vi "Retrieve and visualize_SE.vi"(11 "Field/Temperature":i32(slide) min=0 max=36 step=1 scale=-1.1..1.0) -> (1 "slowest":dbl=-2499.957 format="%#_6p")   [LabVIEW 2020, in "Retrieve and Visualize.lvclass"]
uses:
  Retrieve and Visualize.lvclass
  <vilib>/Analysis/NI_AAL_SigProc.lvlib
  <userlib>/LevyLab/Graph Utilities/graph_utilities.lvclass
  <userlib>/LevyLab/XY Utilities/xy_utilities.lvlib
  <userlib>/LevyLab/XY Utilities/subVIs/Interpolate (single).vi
  <userlib>/LevyLab/XY Utilities/Typedefs/Interpolation Configuration--cluster.ctl
  <userlib>/LevyLab/LV-Data/LV-Data.ITX/LV-Data.ITX.lvclass
  <userlib>/LevyLab/Instrument Framework/SMOs/Configuration/Configuration.lvclass
  typedefs/Choose Intensity Data--enum.ctl
  typedefs/INI--Cluster.ctl
  <vilib>/Utility/sysdir.llb/System Directory Type.ctl
  <userlib>/_OpenG.lib/file/file.llb/File Exists - Scalar__ogtk.vi
  typedefs/IV Setup--Cluster.ctl
  <userlib>/LevyLab/LV-Data/LV-Data/Typedefs/File Type--enum.ctl
  <userlib>/LevyLab/LV-Data/LV-Data/LV-Data.lvclass
panel:
  in  "Window [h] (2)":dbl=2.0
  in  "Interval Units (points)":enum16{"Points", "Data"}(ring)
  in  "Subset Slider (%)":cluster{dbl, dbl}(slide)={75.0, 25.0} scale=0.0..100.0 scale format="%#_6f"
  in  "Export ITX Name":string="B2"
  in  "Export What?":T1(ring)
  in  "Export ITX":bool
  in  "Export ITX Path":path=path "C:/"
  out "Status":string="Exit"
  out "Slow":dbl=88828.125
  out "Fast":dbl=-0.009836065573770498
  in  "OK":bool
  in  "Open DAT Path":path=path "C:/"
  in  "S-G side points (4T)":i32=8
  in  "S-G side points (2T)":i32=12
  in  "Visualize Button":bool
  in  "Tab Control":T2(tab)=enum."Intensity Graphs"
  out "Comments":string
  in  "Check Files Button":bool
  in  "Generate Button":bool
  in  "Additional comments":string
  in  "Field Period":i32=1
  in  "# of fields/Temperatures":i32=1
  in  "Path":path=path "C:/"
  in  "DAT folder":path=path "C:/"
  in  "IV file name":string="Name.dat"
  in  "IV setup":T3={"# Vslow"=11, "# Vfast"=251, "#IV Curves at each gate"=1, "B/T offset"=0, "Discard first # curves"=0, "Manual offset"=0}
  in  "Scan names":string[](array[string])=["appliedVsg", "appliedField", "appliedField"]
  in  "Portion of data (%)":cluster{dbl, dbl}(slide)={1.0, 0.0} scale=0.0..100.0
  in  "Decimate point":dbl=10.0 format="%#_1f"
  in  "Extract paramaters from comments?":bool=TRUE
  in  "index":T4={"A"=7, "B"=6, "C"=3, "D"=6, "E"=3, "N1"=2, "N2"=2, "N3"=3, "N4"=4, "A 1"=8, "A 2"=10, "C 1"=5, "C 2"=1, "E 2"=4}
  in  "T/B third axis":bool
  in  "File Type":T5
  out "IV":cluster{dbl[], dbl[]}[](graph)
  out "dI/dV":cluster{dbl[], dbl[]}[](graph)
  out "dI/dV 2T":cluster{dbl[], dbl[]}[](graph)
  out "IV 2T":cluster{dbl[], dbl[]}[](graph)
  out "dV/dI":cluster{dbl[], dbl[]}[](graph)
  out "dV/dI 2T":cluster{dbl[], dbl[]}[](graph)
  out "IV slow 2T":cluster{dbl[], dbl[]}[](graph)
  out "dI/dV slow 2T":cluster{dbl[], dbl[]}[](graph)
  out "IV slow 4T":cluster{dbl[], dbl[]}[](graph)
  out "dI/dV slow 4T":cluster{dbl[], dbl[]}[](graph)
  out "IV vary 3rd 2T":cluster{dbl[], dbl[]}[](graph)
  out "dI/dV vary 3rd 2T":cluster{dbl[], dbl[]}[](graph)
  out "IV vary 3rd 4T":cluster{dbl[], dbl[]}[](graph)
  out "dI/dV vary 3rd 4T":cluster{dbl[], dbl[]}[](graph)
  in  "fake point 1":dbl format="%#_6p"
  in  "Log scale? 1":bool
  in  "e^2/h? 1":bool=TRUE
  in  "e^2/h? 2":bool=TRUE
  in  "Log scale? 2":bool
  in  "fake point 2":dbl format="%#_6p"
  in  "Intensity 1":T6=enum."G-4T"
  out "Intensity Graph 1":dbl[][](graph)
  out "Intensity Graph 2":dbl[][](graph)
  out "H Cut 1":cluster{dbl[], dbl[]}[](graph)
  out "V Cut 1":cluster{dbl[], dbl[]}[](graph)
  out "H Cut 2":cluster{dbl[], dbl[]}[](graph)
  out "V Cut 2":cluster{dbl[], dbl[]}[](graph)
  in  "Intensity 2":T6=enum."dGdVsg-4T"
  in  "X Offset 1":dbl format="%#_6p"
  in  "X Offset 2":dbl format="%#_6p"
  out "x3D Intensity Graph 11":dbl[][](graph)
  out "x3D Intensity Graph 10":dbl[][](graph)
  out "x3D Intensity Graph 9":dbl[][](graph)
  out "x3D Transconductance 2":dbl[][](graph)
  out "bottom loop":dbl[](graph)
  out "xalpha top loop":dbl[](graph)
  out "xalpha Top loop Intensity Graph":dbl[][](graph)
  out "xalpha Vsd vs Vsg":cluster{dbl[], dbl[]}(graph)
  in  "xalpha threshold 2":dbl format="%0.2f"
  in  "xalpha width 2":i32=3 min=3
  out "xalpha Y line cut 9":cluster{dbl[], dbl[]}[](graph)
  out "xalpha Vsg?":dbl[](array[numeric])
  out "xalpha vertical peak diff":dbl[](array[numeric])
  in  "xalpha threshold":dbl format="%0.2f"
  in  "xalpha width":i32=3 min=3
  in  "xalpha derivative bin size":dbl=10.0
  in  "Diff Interval":dbl=12.0
  in  "derivative bin size 2":dbl=12.0
  in  "derivative bin size 1":dbl=12.0
  in  "SG Filter?":bool=TRUE
  out "Cursor Graph":cluster{dbl[], dbl[]}(graph)
  # "I+"
  # "V+"
  # "Vsg1"
  # "Vsgw"
  # "Vsg2"
  # "V-"
  # "I-"
  # "Input"
  # "Process Parameters"
  # "Vfast"
  # "Vslow"
  # "Vslowest"
  # "obsolete?"
  # "A: V4\nB: I\nC: V2\nD: I\nA1,A2: V4 SE\nC1,C2: V2 SE\n\n#todo: replace with rings"
  # "DOESN'T WORK ANY MORE"
  # "Output"
  # "#todo: add button to automatically populate output and filename fields"
  # "Used??"
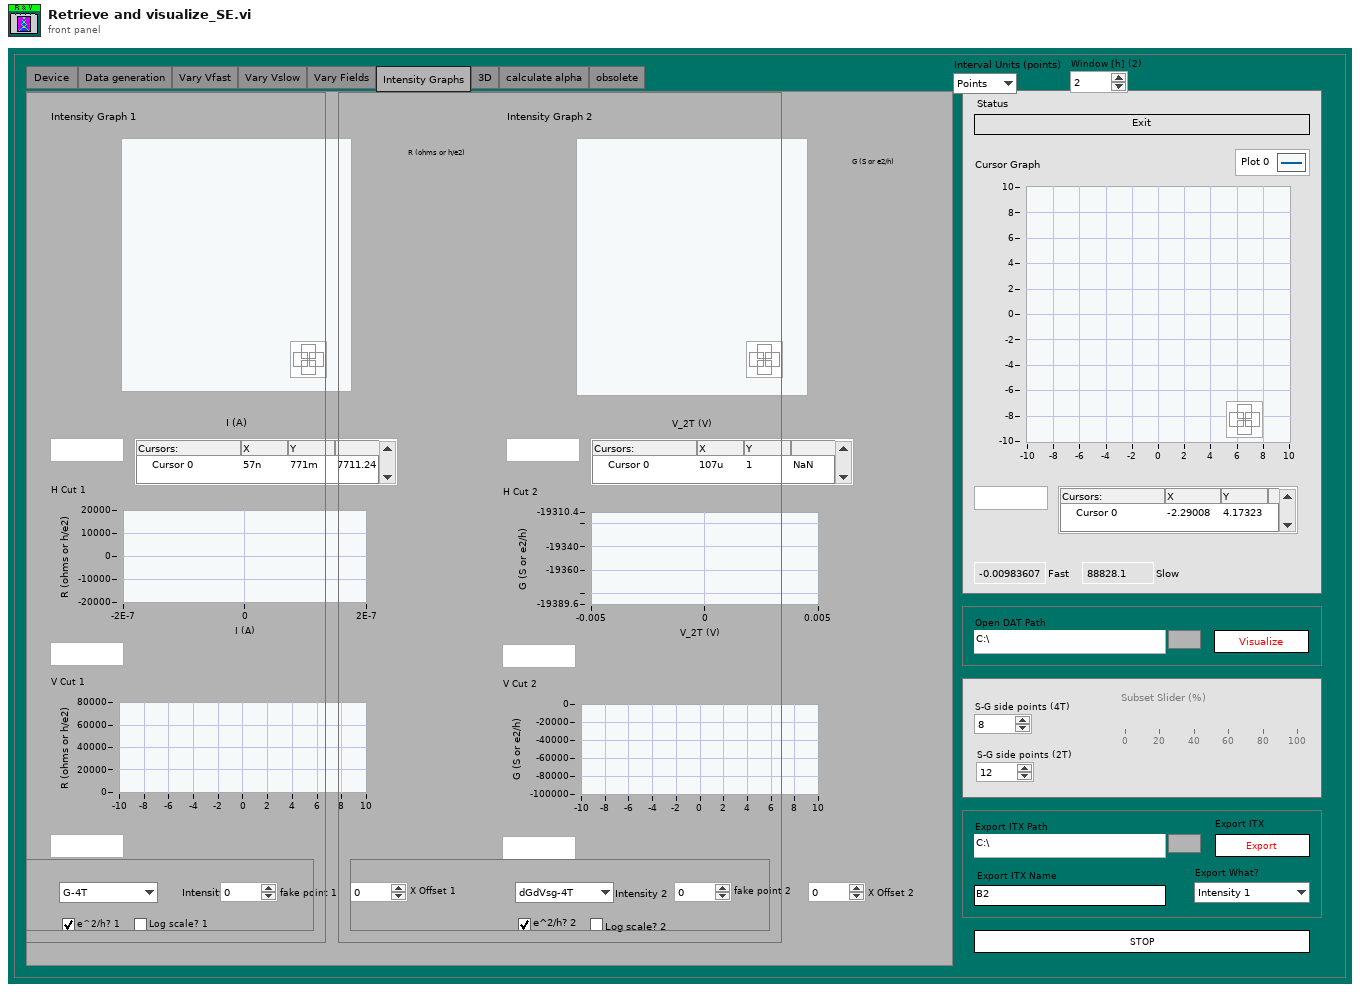
[diagram p1: front panel]
types:
  T1 = enum16{"Intensity 1", "H Cut 1", "V Cut 1", "Intensity 2", "H Cut 2", "V Cut 2"}
  T2 = enum32{"Device ", "Data generation", "Vary Vfast", "Vary Vslow", "Vary Fields", "Intensity Graphs", "3D", "calculate alpha", "obsolete"}
  T3 = typedef "Retrieve and Visualize.lvclass/IV Setup--Cluster.ctl" = cluster{"# Vslow":i32, "# Vfast":i32, "#IV Curves at each gate":i32, "B/T offset":i32, "Discard first # curves":i32, "Manual offset":i32}
  T4 = cluster{"A":i32, "B":i32, "C":i32, "D":i32, "E":i32, "N1":i32, "N2":i32, "N3":i32, "N4":i32, "A 1":i32, "A 2":i32, "C 1":i32, "C 2":i32, "E 2":i32}
  T5 = typedef "LV-Data.lvclass/File Type--enum.ctl" = enum16{"DAT", "ITX", "TDMS", "VI"}
  T6 = typedef "Retrieve and Visualize.lvclass/Choose Intensity Data--enum.ctl" = enum16{"IV-4T", "IV-2T", "R-4T", "G-4T", "R-2T", "G-2T", "dGdVsg-4T", "dGdVsg-2T"}
  T7 = enum32{"Device ", "Data generation", "Vary Vfast", "Vary Vslow", "Vary Fields", "Intensity Graphs", "3D (disabled)", "calculate alpha (disabled)"}
  T8 = cluster{"IV-4T":refnum<data-value>, "G-2T":refnum<data-value>, "R-2T":refnum<data-value>, "G-4T":refnum<data-value>, "R-4T":refnum<data-value>, "IV-2T":refnum<data-value>, "Vfast":dbl[][], "Vslow":dbl[], "Vslowest":dbl[], "Scan Names":string[]}
  T9 = typedef "xy_utilities.lvlib/Interpolation Configuration--cluster.ctl" = cluster{"X Low":dbl, "X High":dbl, "X Step":dbl, "Fake Point":dbl}
  T10 = typedef "LVOffsetAndMultiplierTypeDef.ctl" = cluster{"Offset":dbl, "Multiplier":dbl}
  T11 = enum32{"Invalid", "Standard", "Closed", "Hidden", "Minimized", "Maximized"}
  T12 = enum32{"invalid app kind", "Development System", "Run Time System", "Student Edition", "Embedded LabVIEW", "Evaluation", "Custom"}
  T13 = enum32{"Device ", "Data generation", "Vary Vfast", "Vary Vslow", "Vary Fields", "Intensity Graphs", "3D", "calculate alpha"}
  T14 = cluster{"V2T":string, "V+":string, "V-":string, "I (A)":string, "+X":string, "+Y":string, "-X":string, "-Y":string, "B":string}
  T15 = typedef "Retrieve and Visualize.lvclass/INI--Cluster.ctl" = cluster{"Open DAT Path":path, "Export ITX Path":path, "Export ITX Name":string, "Intensity 1":T6, "X Offset 1":dbl, "derivative bin size 1":dbl, "e^2/h? 1":bool, "Log scale? 1":bool, "fake point 1":dbl, "Intensity 2":T6, "X Offset 2":dbl, "derivative bin size 2":dbl, "e^2/h? 2":bool, "Log scale? 2":bool, "fake point 2":dbl}
  T16 = cluster{"Core":cluster{"Current VI Reference":refnum<vi>, "Close Panel on Exit?":bool}, "Retrieve and Visualize":refnum<class "Retrieve and Visualize.lvclass">, "Configuration":refnum<class "Configuration.lvclass">, "INI":T15, "DVR":cluster{"IV-4T":refnum<data-value>, "IV-2T":refnum<data-value>, "G-4T":refnum<data-value>, "R-4T":refnum<data-value>, "G-2T":refnum<data-value>, "R-2T":refnum<data-value>}, "Graph":cluster{"Intensity 1":refnum<class "graph_utilities.lvclass">, "V 1":refnum<class "graph_utilities.lvclass">, "H 1":refnum<class "graph_utilities.lvclass">, "Intensity 2":refnum<class "graph_utilities.lvclass">, "V 2":refnum<class "graph_utilities.lvclass">, "H 2":refnum<class "graph_utilities.lvclass">}, "Vfast":dbl[][], "Vslow":dbl[], "Vslowest":dbl[], "Scan Names":string[], "Vfast Slice":dbl[], "Vslow Slice":dbl[], "Page":i32, "Row Array":i32[], "Column Array":i32[], "Row":i32, "Column":i32}
  T17 = cluster{"Intensity 1":refnum<class "graph_utilities.lvclass">, "V 1":refnum<class "graph_utilities.lvclass">, "H 1":refnum<class "graph_utilities.lvclass">, "Intensity 2":refnum<class "graph_utilities.lvclass">, "V 2":refnum<class "graph_utilities.lvclass">, "H 2":refnum<class "graph_utilities.lvclass">}
  T18 = cluster{"IV-4T":refnum<data-value>, "IV-2T":refnum<data-value>, "G-4T":refnum<data-value>, "R-4T":refnum<data-value>, "G-2T":refnum<data-value>, "R-2T":refnum<data-value>}
  T19 = cluster{"Current VI Reference":refnum<vi>, "Close Panel on Exit?":bool}
  T20 = typedef "System Directory Type.ctl" = i32
  T21 = typedef "LVPointDoubleTypeDef.ctl" = cluster{"X":dbl, "Y":dbl}
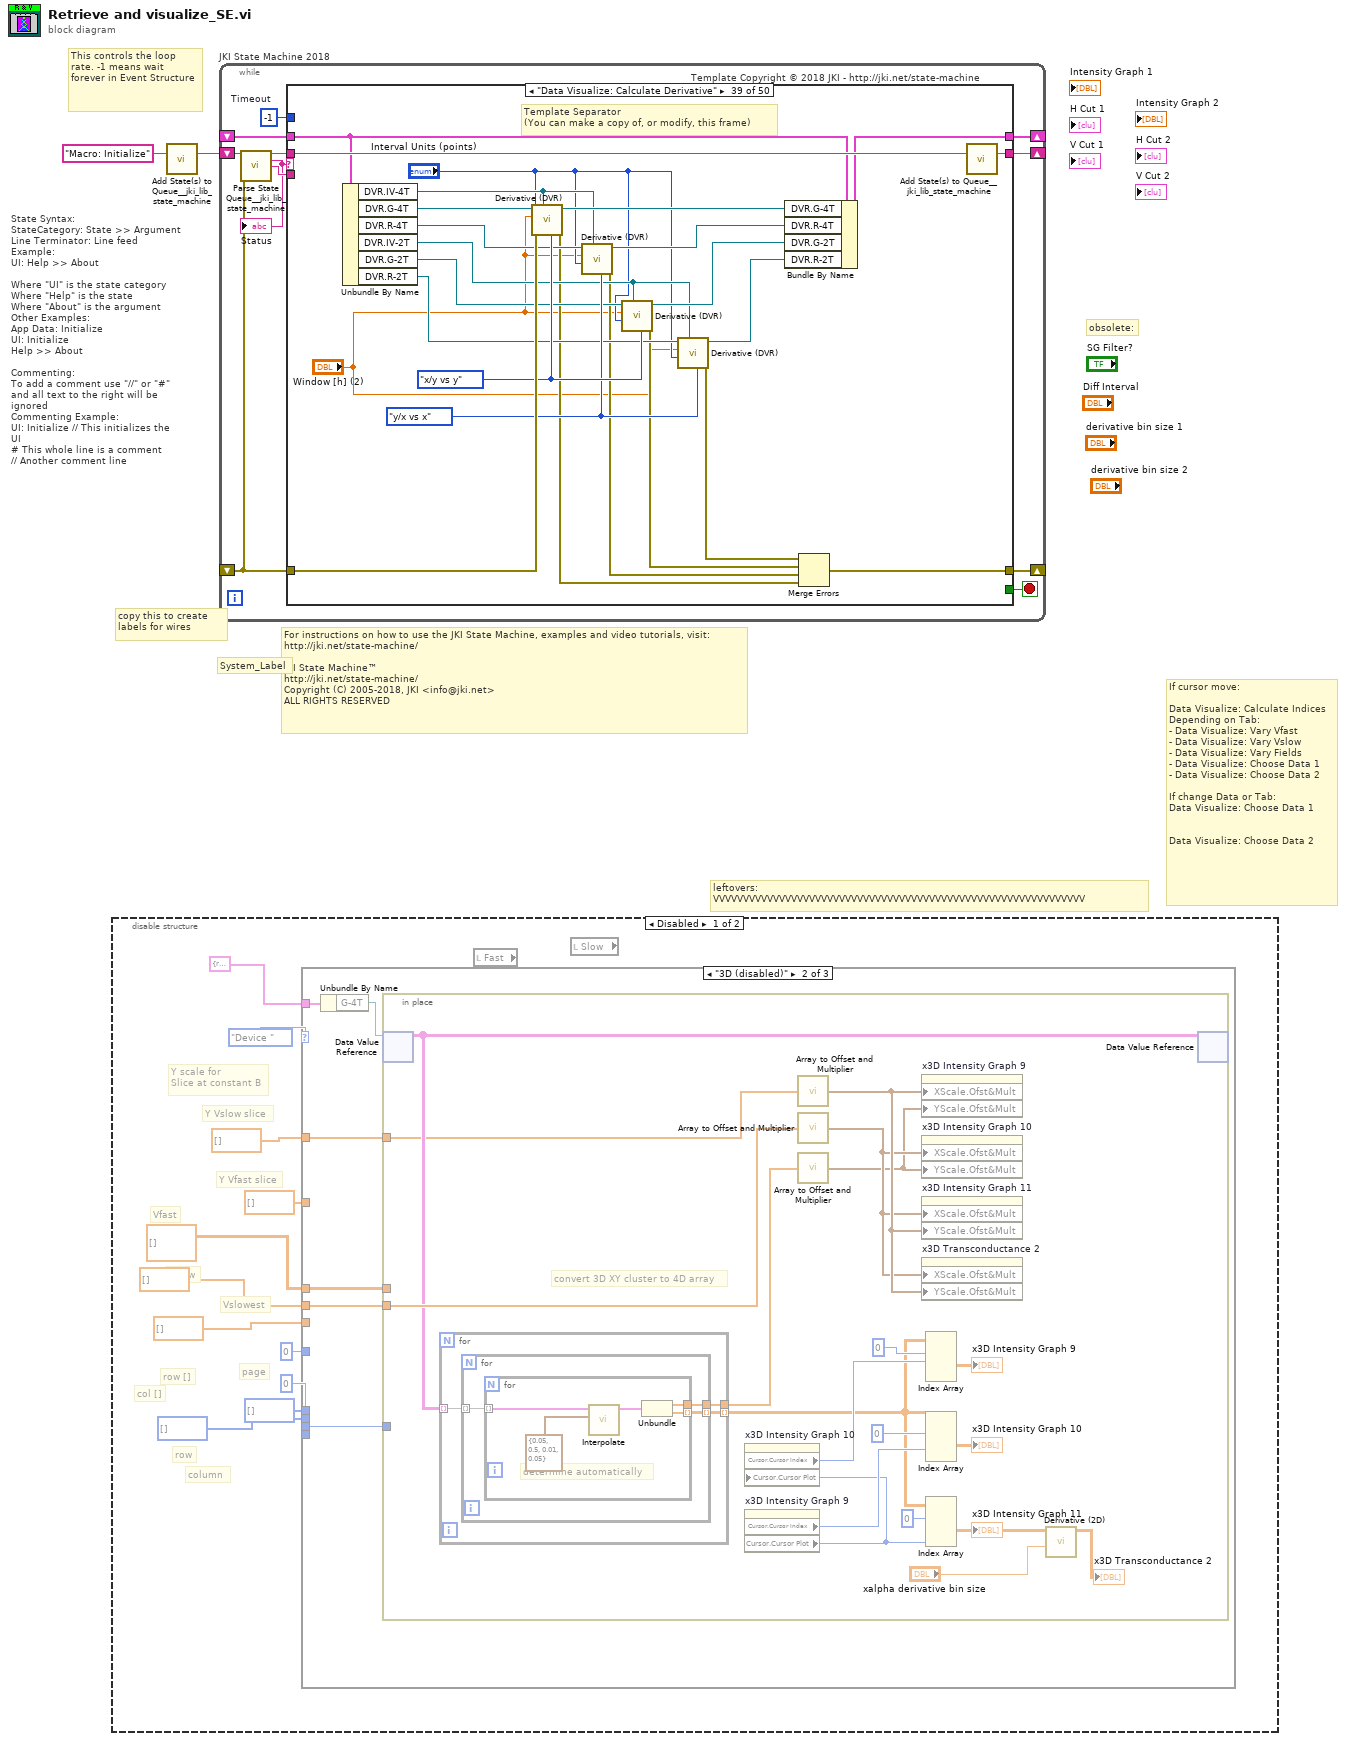
[diagram p0: block diagram]
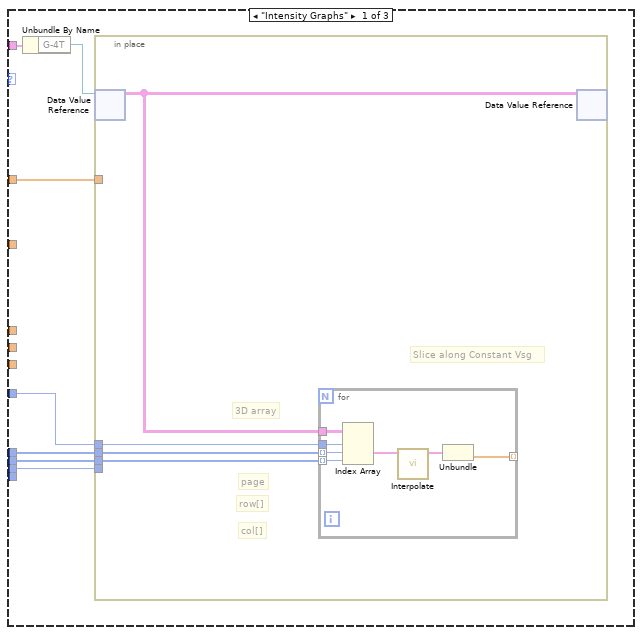
[diagram p2: hidden frame]
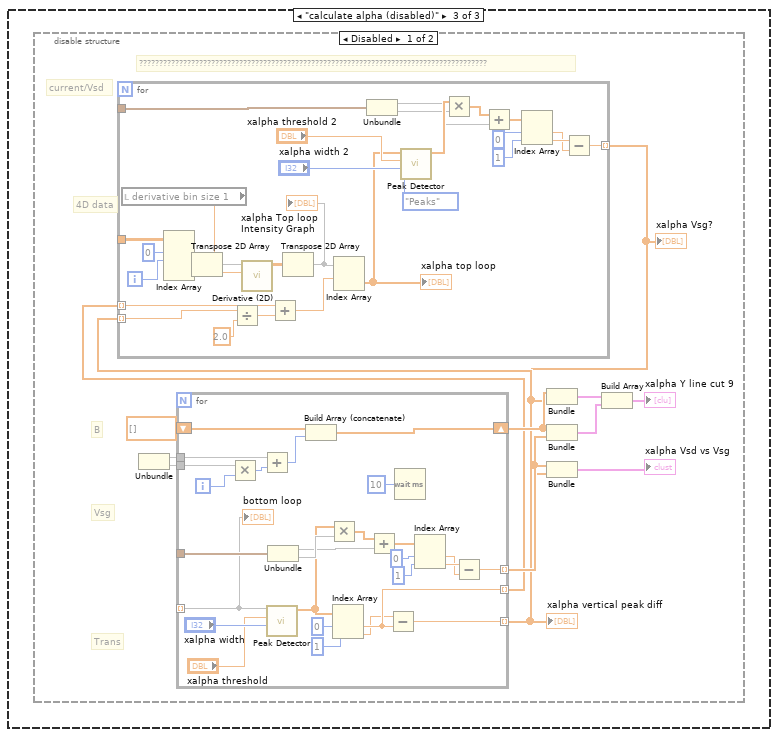
[diagram p3: hidden frame]
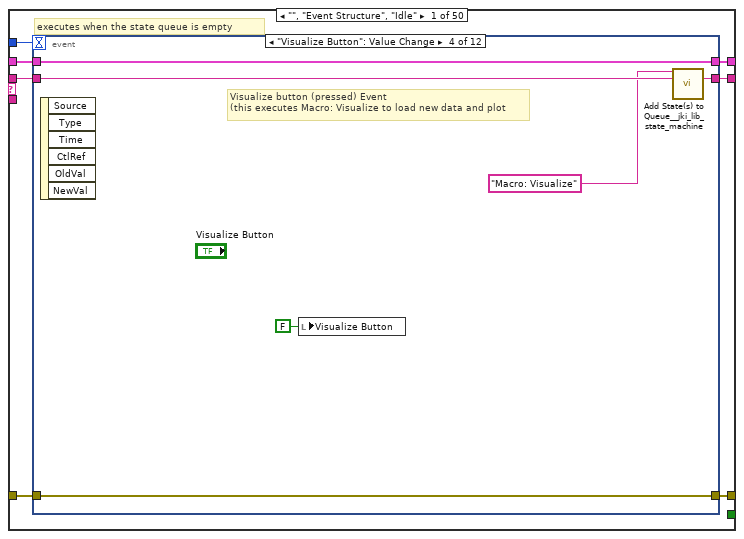
[diagram p6: hidden frame]
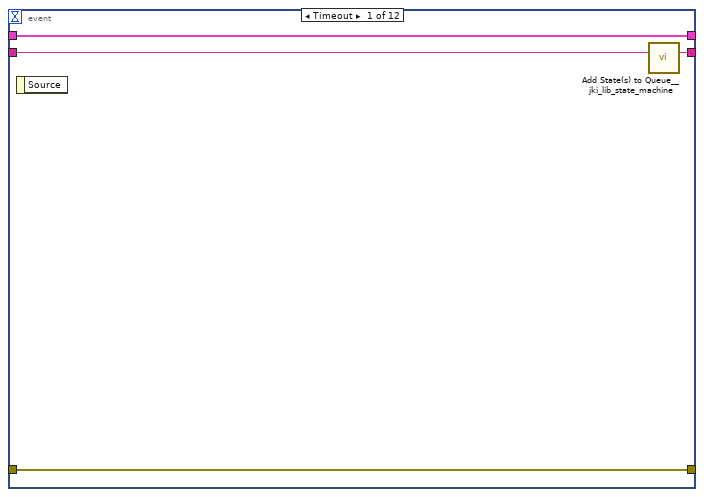
[diagram p7: hidden frame]
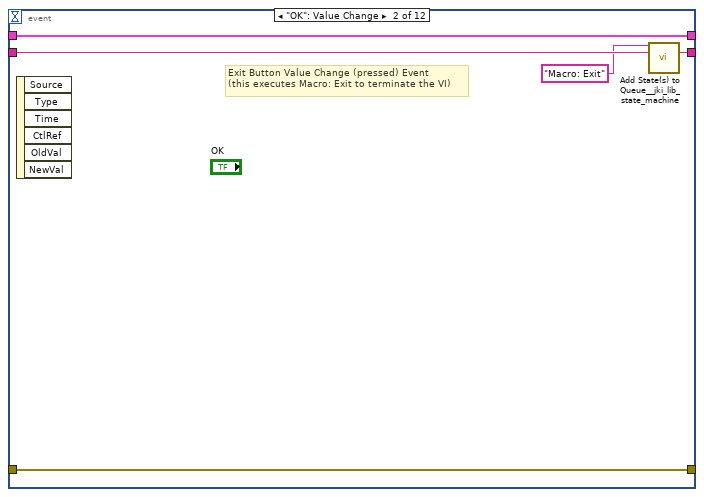
[diagram p8: hidden frame]
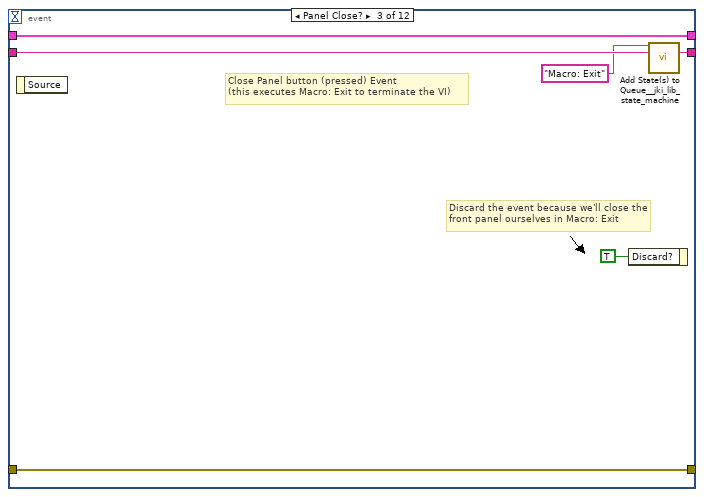
[diagram p9: hidden frame]
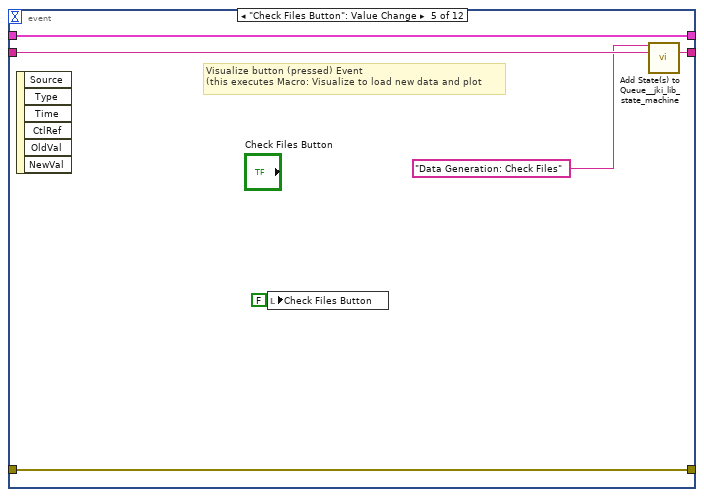
[diagram p10: hidden frame]
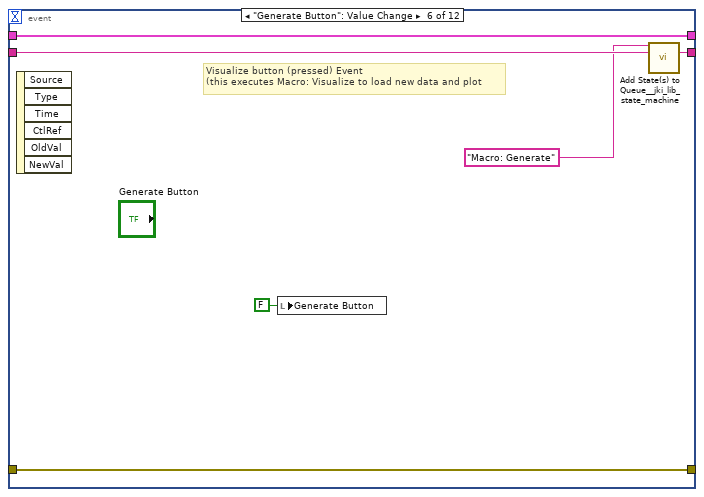
[diagram p11: hidden frame]
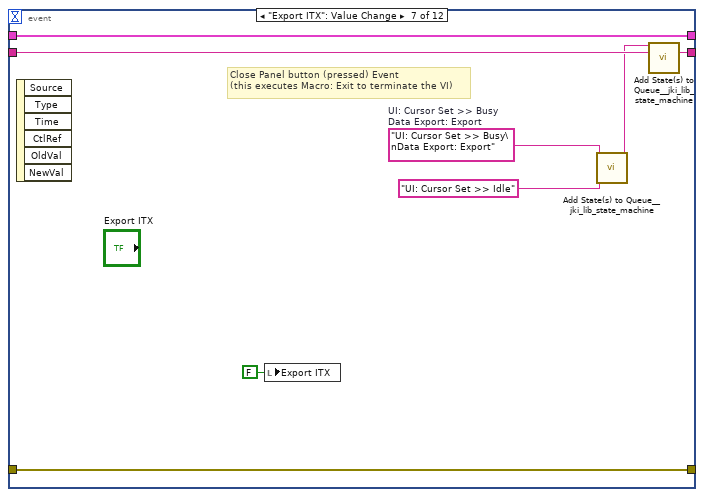
[diagram p12: hidden frame]
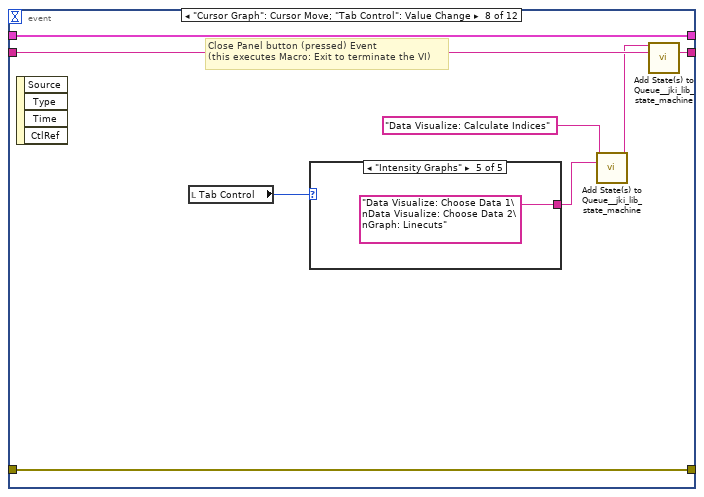
[diagram p13: hidden frame]
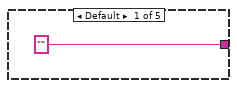
[diagram p14: hidden frame]
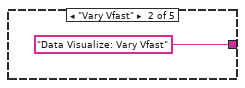
[diagram p15: hidden frame]
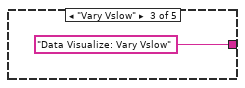
[diagram p16: hidden frame]
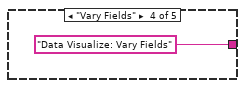
[diagram p17: hidden frame]
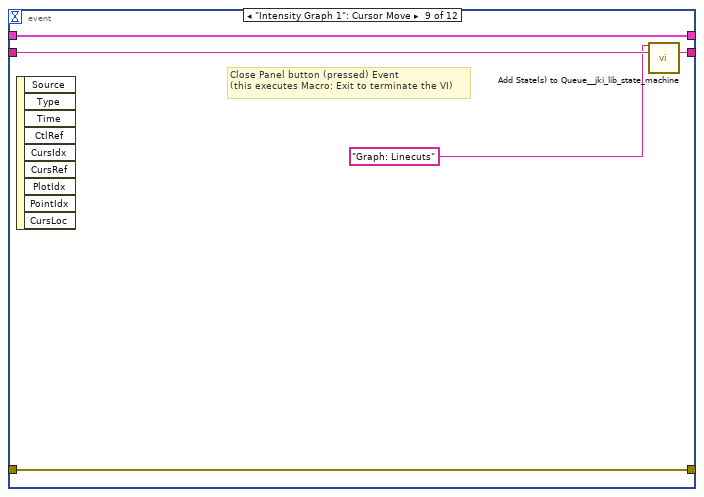
[diagram p18: hidden frame]
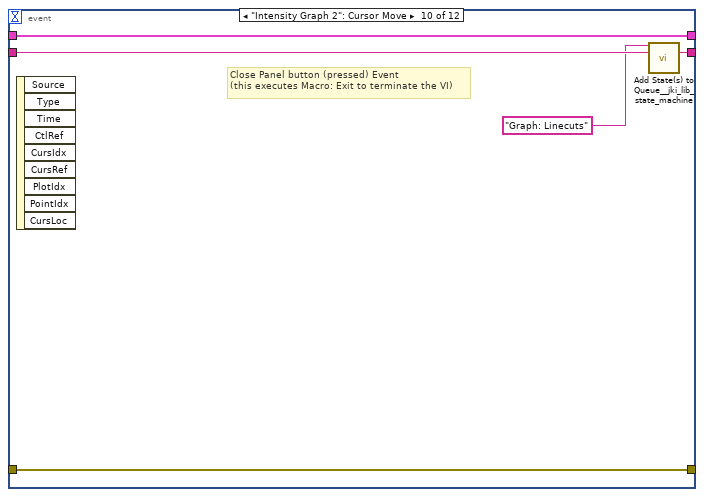
[diagram p19: hidden frame]
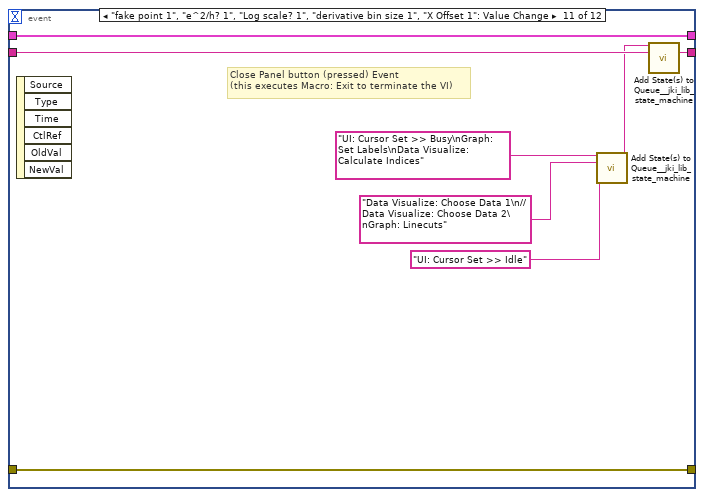
[diagram p20: hidden frame]
diagram:
  # "obsolete:"
  # "If cursor move:\n\nData Visualize: Calculate Indices\nDepending on Tab:\n- Data Visualize: Vary Vfast\n- Data Visualize: Vary Vslow\n- Data Visualize: Vary Fields\n- Data Visualize: Choose Data 1\n- Data Visualize: Choose Data 2\n\nIf change Data or Tab:\nData Visualize: Choose Data 1\n\n\nData Visualize: Choose Data 2"
  # "leftovers:\nVVVVVVVVVVVVVVVVVVVVVVVVVVVVVVVVVVVVVVVVVVVVVVVVVVVVVVVVVVVVVV"
  # "For instructions on how to use the JKI State Machine, examples and video tutorials, visit:\nhttp://jki.net/state-machine/\n\nJKI State Machine™\nhttp://jki.net/state-machine/\nCopyright (C) 2005-2018, JKI <info@jki.net>\nALL RIGHTS RESERVED"
  # "State Syntax:\nStateCategory: State >> Argument\nLine Terminator: Line feed\nExample:\nUI: Help >> About\n\nWhere \"UI\" is the state category\nWhere \"Help\" is the state\nWhere \"About\" is the argument\nOther Examples:\nApp Data: Initialize\nUI: Initialize\nHelp >> About\n\nCommenting:\nTo add a comment use \"//\" or \"#\" and all text to the right will be ignored\nCommenting Example:\nUI: Initialize // This initializes the UI\n# This whole line is a comment\n// Another comment line"
  # "copy this to create labels for wires"
  # "This controls the loop rate. -1 means wait forever in Event Structure"
  # "System_Label"
  n1 = disable-structure shown="Disabled" {
    frame Disabled {
      # "column"
      # "Y Vfast slice"
      # "Y Vslow slice"
      # "Y scale for \nSlice at constant B"
      # "row"
      # "col []"
      # "row []"
      # "page"
      # "Vslowest"
      # "Vslow"
      # "Vfast"
      n2 = case shown="\"3D (disabled)\"" T7."Device " ("Tab Control") {
        tunnel: 0 ("Field/Temperature") -> [w20 _ _]
        tunnel: 0 ("Row") -> [w21 w38 _]
        tunnel: dbl[][] [] ("Vfast") -> [_ w36 _]
        tunnel: dbl[] [] ("Vslow") -> [_ w37 _]
        tunnel: dbl[] [] ("Vslowest") -> [_ _ _]
        tunnel: i32[] [] ("Row Array") -> [w19 _ _]
        tunnel: i32[] [] ("Column Array") -> [w18 _ _]
        tunnel: T8 {"IV-4T"=refnum, "G-2T"=refnum, "R-2T"=refnum, "G-4T"=refnum, "R-4T"=refnum, "IV-2T"=refnum, "Vfast"=[], "Vslow"=[], "Vslowest"=[], "Scan Names"=[]} -> [w15 w35 _]
        tunnel: dbl[] [] ("Vfast") -> [w16 w33 _]
        tunnel: dbl[] [] -> [_ _ _]
        tunnel: 0 ("Column") -> [_ _ _]
        frame "Intensity Graphs" {
          n3 = Unbundle By Name(w15) -> ("G-4T"=w17:refnum<data-value>)
          n4 = in-place {
            in-place-border: w21 -> [_]
            in-place-border: w20 -> [w25]
            in-place-border: w19 -> [w24]
            in-place-border: w18 -> [w23]
            in-place-border: w16 -> [_]
            # "page"
            # "3D array"
            # "row[]"
            # "col[]"
            # "Slice along Constant Vsg"
            n5 = in-place-dvr #1(w17) -> (w22:cluster{dbl[], dbl[]}[][][])  [unwired: 1 out]
            n6 = for {
              tunnel: w22 -> [w32]
              tunnel: w25 -> [w31]
              tunnel: w24 -> [w28] mode=indexing
              tunnel: w23 -> [w29] mode=indexing
              tunnel: [w30] -> _ mode=indexing
              n7 = Index Array(array=w32, index (dim 0)=w31, index (dim 1)=w28, index (dim 2)=w29) -> (element=w27:cluster{dbl[], dbl[]})
              n8 = call-poly <userlib>:"Interpolate.vi"("XY-data"=w27) -> ("Interpolated XY-data out"=w26:cluster{"X-array":dbl[], "Y-array":dbl[]})  [unwired: 9 in, 1 out]
              n9 = Unbundle(w26) -> ("Y-array"=w30:dbl[])  [unwired: 1 out]
            }
            n10 = in-place-dvr #1(w22) -> ()  [unwired: 2 out]
          }
        }
        frame "3D (disabled)" {
          n11 = Unbundle By Name(w35) -> ("G-4T"=w34:refnum<data-value>)
          n12 = in-place {
            in-place-border: w38 -> [_]
            in-place-border: w37 -> [w46]
            in-place-border: w36 -> [_]
            in-place-border: w33 -> [w43]
            # "convert 3D XY cluster to 4D array"
            n13 = in-place-dvr #2(w34) -> (w44:cluster{dbl[], dbl[]}[][][])  [unwired: 1 out]
            n14 = for {
              tunnel: w44 -> [w60] mode=indexing
              tunnel: [w59] -> w49 mode=indexing
              tunnel: [w58] -> w39
              n15 = for {
                tunnel: w60 -> [w63] mode=indexing
                tunnel: [w62] -> w59 mode=indexing
                tunnel: [w61] -> w58
                n16 = for {
                  tunnel: w63 -> [w67] mode=indexing
                  tunnel: [w68] -> w62 mode=indexing
                  tunnel: [w65] -> w61
                  # "determine automatically"
                  n17 = call-poly <userlib>:"Interpolate.vi"("Configure"=T9 {"X Low"=0.05, "X High"=0.5, "X Step"=0.01, "Fake Point"=0.05}, "XY-data"=w67) -> ("Interpolated XY-data out"=w66:cluster{"X-array":dbl[], "Y-array":dbl[]})  [unwired: 8 in, 1 out]
                  n18 = Unbundle(w66) -> ("X-array"=w65:dbl[], "Y-array"=w68:dbl[])
                }
              }
            }
            n19 = property on="x3D Intensity Graph 9" class="IntGraph (strict)"() -> ("Cursor.Cursor Index"=w57:i32, "Cursor.Cursor Plot"=w40:i32)  [unwired: 2 in, 2 out]
            n20 = property on="x3D Intensity Graph 10" class="IntGraph (strict)"("Cursor.Cursor Plot"=w40) -> ("Cursor.Cursor Index"=w56:i32)  [unwired: 2 in, 2 out]
            n21 = call <userlib>:"Array to Offset and Multiplier.vi"("Array"=w43) -> ("Offset and Multiplier"=w47:T10)
            n22 = call <userlib>:"Array to Offset and Multiplier.vi"("Array"=w46) -> ("Offset and Multiplier"=w45:T10)
            n23 = call <userlib>:"Array to Offset and Multiplier.vi"("Array"=w39) -> ("Offset and Multiplier"=w42:T10)
            n24 = property on="x3D Intensity Graph 9" class="IntGraph (strict)"("XScale.Ofst&Mult"=w47, "YScale.Ofst&Mult"=w42) -> ()  [unwired: 2 in, 2 out]
            n25 = property on="x3D Intensity Graph 10" class="IntGraph (strict)"("XScale.Ofst&Mult"=w45, "YScale.Ofst&Mult"=w42) -> ()  [unwired: 2 in, 2 out]
            n26 = property on="x3D Intensity Graph 11" class="IntGraph (strict)"("XScale.Ofst&Mult"=w45, "YScale.Ofst&Mult"=w47) -> ()  [unwired: 2 in, 2 out]
            n27 = property on="x3D Transconductance 2" class="IntGraph (strict)"("XScale.Ofst&Mult"=w45, "YScale.Ofst&Mult"=w47) -> ()  [unwired: 2 in, 2 out]
            n28 = Index Array(array=w49, index (dim 0)=0 ("index (vol)"), index (dim 1)=w56) -> (element=→"x3D Intensity Graph 9":dbl[][])  [unwired: 2 in]
            n29 = Index Array(array=w49, index (dim 0)=0 ("disabled index (page) 2"), index (dim 2)=w57) -> (element=→"x3D Intensity Graph 10":dbl[][])  [unwired: 2 in]
            n30 = Index Array(array=w49, index (dim 0)=0 ("disabled index (row) 2"), index (dim 3)=w40) -> (element=w51:dbl[][])  [unwired: 2 in]
            "x3D Intensity Graph 11" <- w51
            n31 = call "Derivative (2D).vi"("Window [h] (2)"="xalpha derivative bin size", "Conductance"=w51) -> ("Transconductance"=→"x3D Transconductance 2":dbl[][])  [unwired: 7 in, 2 out]
            n32 = in-place-dvr #2(w44) -> ()  [unwired: 2 out]
          }
        }
        frame "calculate alpha (disabled)" {
          n33 = disable-structure shown="Disabled" {
            frame Disabled {
              # "???????????????????????????????????????????????????????????????????????????????????????"
              # "4D data"
              # "Trans"
              # "B"
              # "current/Vsd"
              # "Vsg"
              n34 = Unbundle() -> (w84:T10, "Offset"=w75, "Multiplier"=w74)
              n35 = for {
                tunnel: [w118] -> w85 mode=indexing
                tunnel: [w127] -> w71 mode=indexing
                tunnel: w75 -> [w138]
                tunnel: w74 -> [w137]
                shift-right: [w134] -> w78
                shift-left: dbl[] [] -> [w132]
                tunnel: [w131] -> w72 mode=indexing
                tunnel: [w128] -> w82
                tunnel: [w119] -> w77 mode=indexing
                i -> [w136]
                n36 = Multiply(x=w137, y=w136) -> (x*y=w135:i32)
                n37 = Add(x=w138, y=w135) -> (x+y=w133:i32)
                n38 = call <vilib>:"Peak Detector.vi"("width"="xalpha width", "threshold"="xalpha threshold", "X"=w118) -> ("Locations"=w124:dbl[])  [unwired: 4 in, 4 out]
                n39 = Unbundle(w128) -> ("Offset"=w125, "Multiplier"=w126)
                n40 = Build Array (concatenate)(w132, w133) -> (w134:dbl[])
                n41 = Multiply(x=w124, y=w126) -> (x*y=w129:dbl[])
                n42 = Index Array(array=w124, index #1=0 ("index"), index #2=1 ("index")) -> (element #1=w131:dbl, element #2=w130:dbl)
                n43 = Add(x=w129, y=w125) -> (x+y=w123:dbl[])
                n44 = Subtract(x=w130, y=w131) -> (x-y=w127:dbl)
                n45 = Wait (ms)(milliseconds to wait=u32 10) -> ()  [unwired: 1 out]
                n46 = Index Array(array=w123, index #1=0 ("index"), index #2=1 ("index")) -> (element #1=w120:dbl, element #2=w121:dbl)
                n47 = Subtract(x=w121, y=w120) -> (x-y=w119:dbl)
                "bottom loop" <- w118
              }
              "xalpha vertical peak diff" <- w71
              n48 = for {
                tunnel: [w113] -> w69
                tunnel: w71 -> [w100] mode=indexing
                tunnel: w72 -> [w103] mode=indexing
                tunnel: [w98] -> w83
                tunnel: [w94] -> w70 mode=indexing
                i -> [w111]
                n49 = local read "derivative bin size 1"() -> (w110:dbl)
                n50 = Index Array(array=w113, index (dim 0)=0 ("index (vol)"), index (dim 1)=w111) -> (element=w106)  [unwired: 2 in]
                n51 = Transpose 2D Array(2D array=w106) -> (transposed array=w105:void[][])
                n52 = Divide(x=w100, y=2.0) -> (x/y=w102:dbl)
                n53 = call "Derivative (2D).vi"("Axis Array"=w110, "Conductance"=w105) -> ("Transconductance"=w104:dbl[][])  [unwired: 7 in, 2 out]
                n54 = Add(x=w103, y=w102) -> (x+y=w101:dbl)
                n55 = Transpose 2D Array(2D array=w104) -> (transposed array=w87:dbl[][])
                "xalpha Top loop Intensity Graph" <- w87
                n56 = Index Array(array=w87, index (row)=w101) -> (element=w86:dbl[])  [unwired: 1 in]
                "xalpha top loop" <- w86
                n57 = Unbundle(w98) -> ("Offset"=w92, "Multiplier"=w93)
                n58 = call <vilib>:"Peak Detector.vi"("peaks/valleys"=enum32{"Peaks", "Valleys"}."Peaks", "width"="xalpha width 2", "threshold"="xalpha threshold 2", "X"=w86) -> ("Locations"=w96:dbl[])  [unwired: 3 in, 4 out]
                n59 = Multiply(x=w96, y=w93) -> (x*y=w97:dbl[])
                n60 = Add(x=w97, y=w92) -> (x+y=w95:dbl[])
                n61 = Index Array(array=w95, index #1=0 ("index"), index #2=1 ("index")) -> (element #1=w90:dbl, element #2=w91:dbl)
                n62 = Subtract(x=w91, y=w90) -> (x-y=w94:dbl)
              }
              "xalpha Vsg?" <- w70
              n63 = Bundle(w78, w70) -> (w79:cluster{dbl[], dbl[]})  [unwired: 1 in]
              n64 = Bundle(w78, w77) -> (w81:cluster{dbl[], dbl[]})  [unwired: 1 in]
              n65 = Bundle(w77, w70) -> (→"xalpha Vsd vs Vsg":cluster{dbl[], dbl[]})  [unwired: 1 in]
              n66 = Build Array(w79, w81) -> (→"xalpha Y line cut 9":cluster{dbl[], dbl[]}[])
            }
            frame Enabled {
            }
          }
        }
      }
      n67 = local read "Fast"() -> ()  [unwired: 1 out]
      n68 = local read "Slow"() -> ()  [unwired: 1 out]
    }
    frame Enabled {
    }
  }
  n69 = call <vilib>:"Add State(s) to Queue__jki_lib_state_machine.vi"("State(s) in (\"\")"="Macro: Initialize") -> ("States Out"=w2:string)  [unwired: 14 in]
  n70 = while "JKI State Machine 2018" {
    shift-right: [w145] -> _
    shift-left: _ -> [w144]
    shift-right: [w148] -> _
    shift-left: _ -> [w142]
    shift-right: [w147] -> _
    shift-left: w2 -> [w149]
    stop <- w146 stop-if-true
    w143 = -1  # Timeout
    # "Template Copyright © 2018 JKI - http://jki.net/state-machine"
    n71 = call <vilib>:"Parse State Queue__jki_lib_state_machine.vi"("State Queue"=w149, "Error In (no error)"=w142) -> ("Remaining States"=w151:string, "Current State"=w141:string, "Arguments"=w150:string)  [unwired: 11 in]
    "Status" <- w141
    n72 = case shown="\"Data Visualize: Calculate Derivative\"" w141 {
      selector: w141 -> [_ _ w243 _ _ _ _ _ _ _ _ _ _ _ _ _ _ _ _ _ _ w540 _ _ _ _ _ _ _ _ _ _ _ _ _ _ _ _ _ _ _ _ _ _ _ _ _ _ _ _]
      tunnel: w151 -> [w158 w242 w247 w266 w267 w276 w280 w301 w307 w325 w348 w352 w375 w392 w409 w422 w426 w436 w456 w462 w473 w544 w552 w557 w568 w572 w577 w582 w586 w601 w610 w627 w640 w644 w660 w693 w711 w727 w757 w771 w791 w803 w825 w837 w867 w900 w937 w985 w1010 w1019]
      tunnel: w150 -> [_ _ _ _ _ _ _ _ _ _ _ _ _ _ _ _ _ _ _ w457 w467 _ _ _ _ _ _ _ _ _ _ _ _ _ _ _ _ _ _ _ _ _ _ _ _ _ _ _ _ _]
      tunnel: w144 -> [w156 w239 w245 w259 w269 w274 w277 _ w302 w310 w331 w349 w373 w390 w406 w420 w423 w429 w438 w460 w469 w541 w549 w554 w565 w569 w574 w579 w583 w594 w607 w624 w636 w641 w656 w689 w698 w714 w755 w767 w789 w801 w814 w828 w860 w893 w935 w983 w1007 w1017]
      tunnel: [w155 w240 w249 w263 errorcluster {"status"=FALSE, "code"=0, "source"=""} ("error out") w273 w278 w298 w303 w318 w327 w350 w360 w379 w407 w410 w424 w431 w454 w458 w470 w542 w550 w555 w566 w570 w575 w580 w584 w599 w603 w625 w637 w642 w658 w681 w696 w725 w736 w760 w787 w799 w804 w835 w865 w898 w917 w966 w1008 w1015] -> w148
      tunnel: w142 -> [w154 w240 w248 w263 w268 w273 w278 w298 w304 w322 w328 w350 _ w385 w407 w411 w424 w432 w454 w459 w471 w542 w550 w555 w566 w570 w575 w580 w584 w599 w604 w625 w638 w642 w646 w682 _ w725 w749 w764 w780 w794 w805 w835 w865 w898 w915 w964 w1008 w1013]
      tunnel: [w157 w241 w246 w265 w271 w275 w279 w300 w306 w324 w347 w351 w374 w391 w408 w421 w425 w435 w455 w461 w472 w543 w551 w556 w567 w571 w576 w581 w585 w600 w609 w626 w639 w643 w659 w692 w710 w726 w756 w770 w790 w802 w824 w836 w866 w899 w936 w984 w1009 w1018] -> w147
      tunnel: [_ _ _ _ _ TRUE _ _ _ _ _ _ _ _ _ _ _ _ _ _ _ _ _ _ _ _ _ _ _ _ _ _ _ _ _ _ _ _ _ _ _ _ _ _ _ _ _ _ _ _] -> w146
      tunnel: [w153 w239 w245 w264 w269 w274 w277 w299 w302 w317 w331 w349 w372 w390 w406 w420 w423 w429 w438 w460 w469 w541 w549 w554 w565 w569 w574 w579 w583 w593 w606 w624 w636 w641 w655 w688 w698 w714 w754 w766 w788 w800 w813 w828 w860 w893 w935 w983 w1007 w1017] -> w145
      tunnel: w143 -> [w152 _ _ _ _ _ _ _ _ _ _ _ _ _ _ _ _ _ _ _ _ _ _ _ _ _ _ _ _ _ _ _ _ _ _ _ _ _ _ _ _ _ _ _ _ _ _ _ _ _]
      frame "", "Event Structure", "Idle" {
        # "executes when the state queue is empty"
        n73 = event shown="[3] \"Visualize Button\": Value Change" {
          selector: _ -> [_ _ _ _ _ _ _ _ _ _ _ _]
          dyn-events: _ -> [_ _ _ _ _ _ _ _ _ _ _ _]
          timeout: w152 -> [_ _ _ _ _ _ _ _ _ _ _ _]
          tunnel: w158 -> [w162 w167 w173 w179 w185 w191 w199 w207 w217 w222 w230 w238]
          tunnel: [w161 w166 w172 w178 w184 w190 w198 w206 w216 w221 w229 w237] -> w157
          tunnel: w156 -> [w159 w164 w170 w176 w182 w188 w196 w204 w214 w219 w227 w235]
          tunnel: [w160 w165 w171 w177 w183 w189 w197 w205 w215 w220 w228 w236] -> w155
          tunnel: w154 -> [w160 w165 w171 w177 w183 w189 w197 w205 w215 w220 w228 w236]
          tunnel: [w159 w164 w170 w176 w182 w188 w196 w204 w214 w219 w227 w235] -> w153
          event Timeout {
            n74 = event-data() -> ()  [unwired: 1 in, 1 out]
            n75 = call <vilib>:"Add State(s) to Queue__jki_lib_state_machine.vi"("State(s) in (\"\")"=w162) -> ("States Out"=w161:string)  [unwired: 14 in]
          }
          event "OK": Value Change {
            # "Exit Button Value Change (pressed) Event\n(this executes Macro: Exit to terminate the VI)"
            n76 = event-data() -> ()  [unwired: 1 in, 6 out]
            n77 = call <vilib>:"Add State(s) to Queue__jki_lib_state_machine.vi"("State(s) in Front (\"\")"="Macro: Exit", "State(s) in (\"\")"=w167) -> ("States Out"=w166:string)  [unwired: 13 in]
          }
          event Panel Close? {
            # "Discard the event because we'll close the front panel ourselves in Macro: Exit"
            # "Close Panel button (pressed) Event\n(this executes Macro: Exit to terminate the VI)"
            n78 = event-data() -> ()  [unwired: 1 in, 1 out]
            n79 = event-data("Discard?"=TRUE) -> ()  [unwired: 1 in, 1 out]
            n80 = call <vilib>:"Add State(s) to Queue__jki_lib_state_machine.vi"("State(s) in Front (\"\")"="Macro: Exit", "State(s) in (\"\")"=w173) -> ("States Out"=w172:string)  [unwired: 13 in]
          }
          event "Visualize Button": Value Change {
            # "Visualize button (pressed) Event\n(this executes Macro: Visualize to load new data and plot"
            n81 = event-data() -> ()  [unwired: 1 in, 6 out]
            n82 = local write "Visualize Button"(FALSE ("Visualize Button")) -> ()
            n83 = call <vilib>:"Add State(s) to Queue__jki_lib_state_machine.vi"("State(s) in Front (\"\")"="Macro: Visualize", "State(s) in (\"\")"=w179) -> ("States Out"=w178:string)  [unwired: 13 in]
          }
          event "Check Files Button": Value Change {
            # "Visualize button (pressed) Event\n(this executes Macro: Visualize to load new data and plot"
            n84 = event-data() -> ()  [unwired: 1 in, 6 out]
            n85 = local write "Check Files Button"(FALSE ("Visualize Button")) -> ()
            n86 = call <vilib>:"Add State(s) to Queue__jki_lib_state_machine.vi"("State(s) in Front (\"\")"="Data Generation: Check Files", "State(s) in (\"\")"=w185) -> ("States Out"=w184:string)  [unwired: 13 in]
          }
          event "Generate Button": Value Change {
            # "Visualize button (pressed) Event\n(this executes Macro: Visualize to load new data and plot"
            n87 = event-data() -> ()  [unwired: 1 in, 6 out]
            n88 = local write "Generate Button"(FALSE ("Generate Button")) -> ()
            n89 = call <vilib>:"Add State(s) to Queue__jki_lib_state_machine.vi"("State(s) in Front (\"\")"="Macro: Generate", "State(s) in (\"\")"=w191) -> ("States Out"=w190:string)  [unwired: 13 in]
          }
          event "Export ITX": Value Change {
            w195 = "UI: Cursor Set >> Busy\nData Export: Export"  # UI: Cursor Set >> Busy Data Export: Export
            # "Close Panel button (pressed) Event\n(this executes Macro: Exit to terminate the VI)"
            n90 = event-data() -> ()  [unwired: 1 in, 6 out]
            n91 = local write "Export ITX"(FALSE ("Export")) -> ()
            n92 = call <vilib>:"Add State(s) to Queue__jki_lib_state_machine.vi"("State(s) in Front (\"\")"=w195, "State(s) at Back (\"\")"="UI: Cursor Set >> Idle") -> ("States Out"=w194:string)  [unwired: 13 in]
            n93 = call <vilib>:"Add State(s) to Queue__jki_lib_state_machine.vi"("State(s) in Front (\"\")"=w194, "State(s) in (\"\")"=w199) -> ("States Out"=w198:string)  [unwired: 13 in]
          }
          event "Cursor Graph": Cursor Move; "Tab Control": Value Change {
            # "Close Panel button (pressed) Event\n(this executes Macro: Exit to terminate the VI)"
            n94 = event-data() -> ()  [unwired: 1 in, 4 out]
            n95 = local read "Tab Control"() -> (w203:T2)
            n96 = case shown="\"Intensity Graphs\"" w203 {
              tunnel: ["" "Data Visualize: Vary Vfast" "Data Visualize: Vary Vslow" "Data Visualize: Vary Fields" "Data Visualize: Choose Data 1\nData Visualize: Choose Data 2\nGraph: Linecuts"] -> w200
              frame Default {
              }
              frame "Vary Vfast" {
              }
              frame "Vary Vslow" {
              }
              frame "Vary Fields" {
              }
              frame "Intensity Graphs" {
              }
            }
            n97 = call <vilib>:"Add State(s) to Queue__jki_lib_state_machine.vi"("State(s) in Front (\"\")"="Data Visualize: Calculate Indices", "State(s) in (\"\")"=w200) -> ("States Out"=w201:string)  [unwired: 13 in]
            n98 = call <vilib>:"Add State(s) to Queue__jki_lib_state_machine.vi"("State(s) in Front (\"\")"=w201, "State(s) in (\"\")"=w207) -> ("States Out"=w206:string)  [unwired: 13 in]
          }
          event "Intensity Graph 1": Cursor Move {
            # "Close Panel button (pressed) Event\n(this executes Macro: Exit to terminate the VI)"
            n99 = event-data() -> ()  [unwired: 1 in, 9 out]
            n100 = call <vilib>:"Add State(s) to Queue__jki_lib_state_machine.vi"("State(s) in Front (\"\")"="Graph: Linecuts", "State(s) in (\"\")"=w217) -> ("States Out"=w216:string)  [unwired: 13 in]
          }
          event "Intensity Graph 2": Cursor Move {
            # "Close Panel button (pressed) Event\n(this executes Macro: Exit to terminate the VI)"
            n101 = event-data() -> ()  [unwired: 1 in, 9 out]
            n102 = call <vilib>:"Add State(s) to Queue__jki_lib_state_machine.vi"("State(s) in Front (\"\")"="Graph: Linecuts", "State(s) in (\"\")"=w222) -> ("States Out"=w221:string)  [unwired: 13 in]
          }
          event "fake point 1", "e^2/h? 1", "Log scale? 1", "derivative bin size 1", "X Offset 1": Value Change {
            # "Close Panel button (pressed) Event\n(this executes Macro: Exit to terminate the VI)"
            n103 = event-data() -> ()  [unwired: 1 in, 6 out]
            n104 = call <vilib>:"Add State(s) to Queue__jki_lib_state_machine.vi"("State(s) in Front (\"\")"="UI: Cursor Set >> Busy\nGraph: Set Labels\nData Visualize: Calculate Indices", "State(s) in (\"\")"="Data Visualize: Choose Data 1\n//Data Visualize: Choose Data 2\nGraph: Linecuts", "State(s) at Back (\"\")"="UI: Cursor Set >> Idle") -> ("States Out"=w225:string)  [unwired: 12 in]
            n105 = call <vilib>:"Add State(s) to Queue__jki_lib_state_machine.vi"("State(s) in Front (\"\")"=w225, "State(s) in (\"\")"=w230) -> ("States Out"=w229:string)  [unwired: 13 in]
          }
          event "fake point 2", "e^2/h? 2", "Log scale? 2", "derivative bin size 2", "X Offset 2": Value Change {
            # "Close Panel button (pressed) Event\n(this executes Macro: Exit to terminate the VI)"
            n106 = event-data() -> ()  [unwired: 1 in, 6 out]
            n107 = call <vilib>:"Add State(s) to Queue__jki_lib_state_machine.vi"("State(s) in Front (\"\")"="UI: Cursor Set >> Busy\nGraph: Set Labels\nData Visualize: Calculate Indices", "State(s) in (\"\")"="//Data Visualize: Choose Data 1\nData Visualize: Choose Data 2\nGraph: Linecuts", "State(s) at Back (\"\")"="UI: Cursor Set >> Idle") -> ("States Out"=w233:string)  [unwired: 12 in]
            n108 = call <vilib>:"Add State(s) to Queue__jki_lib_state_machine.vi"("State(s) in Front (\"\")"=w233, "State(s) in (\"\")"=w238) -> ("States Out"=w237:string)  [unwired: 13 in]
          }
        }
      }
      frame "---------- Core ----------" {
        # "Do not put any code in this frame.\n(it is a separator no-op)"
        n109 = call <vilib>:"Add State(s) to Queue__jki_lib_state_machine.vi"("State(s) in (\"\")"=w242) -> ("States Out"=w241:string)  [unwired: 14 in]
      }
      frame Default {
        w252 = 42 items=["No error", "Argument error", "Memory is full", "Out of zone", "End of file", "File already open", "Generic file I/O error", "File not found", "File permission error", "Disk is full", "Duplicate path", "Too many files open", "System feature not enabled", "Resource file not found", "Cannot add resource", "Resource not found", "Image not found", "Image memory error", "Pen does not exist", "Config type invalid", "Config token not found", "Config parse error", "Config memory error", "Bad external code format", "Bad external code offset", "External code not present", "Null window", "Destroy window error", "Null menu", "Print aborted", "Bad print record", "Print driver error", "Windows error during printing", "Memory error during printing", "Print dialog error", "Generic print error", "Invalid device refnum", "Device not found", "Device parameter error", "Device unit error", "Cannot open device", "Device call aborted", "Generic error", "Cancelled by user", "Object ID too low", "Object ID too high", "Object not in heap", "Unknown heap", "Unknown object (invalid DefProc)", "Unknown object (DefProc not in table)", "Message out of range", "Invalid (null) method", "Unknown message", "Manager call not supported", "Bad address", "Network operation in progress", "Network operation timed out", "Connection is busy", "Network attribute not supported", "Network error", "Address in use", "System out of memory", "Connection aborted", "Connection refused", "Not connected", "Already connected", "Connection closed", "Initialization error (interapplication manager)", "Bad occurrence", "Wait on unbound occurrence handler", "Occurrence queue overflow", "Datalog type conflict", "Unused", "Unrecognized type (interapplication manager)", "Memory corrupt", "Failed to make temporary DLL", "Old CIN version", "Drag socket not found", "Failed to load drop-object", "Failed to register OLE object", "Failed to release OLE object", "Format specifier type mismatch", "Unknown format specifier", "Too few format specifiers", "Too many format specifiers", "Scan failed", "Newer CIN version", "Error converting to variant", "Runtime menu error", "Password tampered", "Variant attribute not found", "Incompatible variant data type", "Event data is not available", "Event Store is not present", "Occurrence is not found", "Event Queue is not created", "Event info is not available", "Refnum passed is NULL", "Error retrieving Class GUID", "Error retrieving CoClass GUID", "Error retrieving TypeLib GUID.", "Bad built application magic bytes.", "Specific driver is different from the specific driver associated with the Logical Name.", "There is no session opened to the class driver.", "Max Error", "MAX - Error with config objects", "MAX - Error loading configuration", "MAX - Group not supported"]
        # "Current State"
        # "Do not delete, rename, or modify this frame.\n(this is used to capture unhandled states and typos)"
        # "Handle mistyped state name (developer tool)"
        n110 = Format Into String(format string="Software Exception: Unhandled State \"%s\"." ("message"), error in=w248, w243) -> (resulting string=w251:string, error out=w250:errorcluster)  [unwired: 1 in]
        n111 = call <vilib>:"Error Cluster From Error Code.vi"("show call chain? (False)"=TRUE, "error in (no error)"=w250, "error message (\"\")"=w251, "error code (0)"=w252) -> ("error out"=w249:errorcluster)  [unwired: 5 in]
        n112 = call <vilib>:"Add State(s) to Queue__jki_lib_state_machine.vi"("State(s) in (\"\")"=w247) -> ("States Out"=w246:string)  [unwired: 14 in]
      }
      frame "Initialize Core Data" {
        # "Do not delete, rename, or modify this frame.\n(this is used to determine panel behavior on exit)"
        # "originally closed?"
        # "exe?"
        # "If panel starts closed or is an EXE, then close it when we exit"
        n113 = property class="VI"() -> ("FP.State"=w256:T11)  [unwired: 2 in, 2 out]
        n114 = property class="App"() -> ("App.Kind"=w262:T12)  [unwired: 2 in, 2 out]
        n115 = control-ref of="Current VI Reference"() -> (w257:refnum<vi>)
        n116 = Equal?(x=w256, y=T11."Closed" ("Front Panel Window:State")) -> (x = y?=w254:bool)
        n117 = Equal?(x=w262, y=T12."Run Time System" ("Application:Kind")) -> (x = y?=w260:bool)
        n118 = Or(x=w254, y=w260) -> (x .or. y?=w258:bool)
        n119 = Bundle By Name(cluster=w259, "Core.Current VI Reference"=w257, "Core.Close Panel on Exit?"=w258) -> (w264:T16)
        n120 = call <vilib>:"Add State(s) to Queue__jki_lib_state_machine.vi"("State(s) in (\"\")"=w266) -> ("States Out"=w265:string)  [unwired: 14 in]
      }
      frame "Error Handler" {
        (unwired) "/* Post Error States"
        # "continue after error"
        # "Unhandled Error -- Display it"
        # "Handle any errors here.\nYou can also output any states to clean-up after errors occur"
        # "Clear error"
        n121 = call <vilib>:"General Error Handler.vi"("error in (no error)"=w268) -> ()  [unwired: 10 in, 5 out]
        n122 = call <vilib>:"Add State(s) to Queue__jki_lib_state_machine.vi"("State(s) in (\"\")"=w267) -> ("States Out"=w271:string)  [unwired: 14 in]
      }
      frame "Exit" {
        # "Do not put any code in this frame.\n(No errors that occur here will be handled.)"
        n123 = call <vilib>:"Add State(s) to Queue__jki_lib_state_machine.vi"("State(s) in (\"\")"=w276) -> ("States Out"=w275:string)  [unwired: 14 in]
      }
      frame "---------- Data ----------" {
        # "Do not put any code in this frame.\n(It is a separator no-op. You can make a copy of this frame to create a new Data frame)"
        n124 = call <vilib>:"Add State(s) to Queue__jki_lib_state_machine.vi"("State(s) in (\"\")"=w280) -> ("States Out"=w279:string)  [unwired: 14 in]
      }
      frame "Data: Initialize" {
        w281 = T15 {"Open DAT Path"=path "", "Export ITX Path"=path "", "Export ITX Name"="", "Intensity 1"=enum."IV-4T", "X Offset 1"=0.0, "derivative bin size 1"=0.0, "e^2/h? 1"=FALSE, "Log scale? 1"=FALSE, "fake point 1"=0.0, "Intensity 2"=enum."IV-4T", "X Offset 2"=0.0, "derivative bin size 2"=0.0, "e^2/h? 2"=FALSE, "Log scale? 2"=FALSE, "fake point 2"=0.0}  # INI
        w282 = refnum<class "Configuration.lvclass"> refnum  # Configuration
        w283 = T17 {"Intensity 1"=refnum, "V 1"=refnum, "H 1"=refnum, "Intensity 2"=refnum, "V 2"=refnum, "H 2"=refnum}  # Graph
        w284 = 0  # Column
        w289 = dbl[] []  # Vslow Slice
        w290 = dbl[] []  # Vfast Slice
        w285 = 0  # Row
        w286 = i32[] []  # Column Array
        w287 = i32[] []  # Row Array
        w288 = 0  # Page
        w291 = T18 {"IV-4T"=refnum, "IV-2T"=refnum, "G-4T"=refnum, "R-4T"=refnum, "G-2T"=refnum, "R-2T"=refnum}  # DVR
        w292 = string[] []  # Scan Names
        w293 = dbl[] []  # Vslowest
        w294 = dbl[] []  # Vslow
        w295 = dbl[][] []  # Vfast
        w296 = refnum<class "Retrieve and Visualize.lvclass"> refnum  # Retrieve and Visualize
        w297 = T19 {"Current VI Reference"=refnum, "Close Panel on Exit?"=FALSE}  # Core
        # "Initialize the shift-register data, here.\n(data names are defined by what you wire into the bundle function)"
        n125 = Bundle("Core"=w297, "Retrieve and Visualize"=w296, "Configuration"=w282, "INI"=w281, "DVR"=w291, "Graph"=w283, "Vfast"=w295, "Vslow"=w294, "Vslowest"=w293, "Scan Names"=w292, "Vfast Slice"=w290, "Vslow Slice"=w289, "Page"=w288, "Row Array"=w287, "Column Array"=w286, "Row"=w285, "Column"=w284) -> (w299:T16)  [unwired: 1 in]
        n126 = call <vilib>:"Add State(s) to Queue__jki_lib_state_machine.vi"("State(s) in (\"\")"=w301) -> ("States Out"=w300:string)  [unwired: 14 in]
      }
      frame "Data: Cleanup" {
        # "Cleanup any data and references, here.\n(this is called automatically, by the Macro: Exit)"
        n127 = Unbundle By Name(w302) -> ("Core.Current VI Reference"=w305:refnum<vi>)
        n128 = Close Reference(reference=w305, error in (no error)=w304) -> (error out=w303:errorcluster)
        n129 = call <vilib>:"Add State(s) to Queue__jki_lib_state_machine.vi"("State(s) in (\"\")"=w307) -> ("States Out"=w306:string)  [unwired: 14 in]
      }
      frame "Data: Read INI" {
        w315 = T20 3 items=["User Home"=0, "User Desktop"=1, "User Documents"=2, "User Application Data"=3, "User Preferences"=4, "User Temporary"=5, "Public Documents"=6, "Public Application Data"=7, "Public Preferences"=8, "Public Cache"=13, "System Core Libraries"=9, "System Installed Libraries"=10, "Application Files"=11, "Boot Volume Root"=12] ("system directory type")
        # "Do not put any code in this frame.\n(It is a separator no-op. You can make a copy of this frame to create a new Data frame)"
        n130 = Unbundle By Name(w310) -> ("Configuration"=w308:refnum<class "Configuration.lvclass">, "INI"=w309:T15)
        n131 = call <vilib>:"Get System Directory.vi"("system directory type"=w315) -> ("system directory"=w312:path)  [unwired: 10 in]
        n132 = Build Path(base path=w312, name or relative path="LevyLab\\Retrieve and Visualize") -> (appended path=w314:path)
        n133 = call <userlib>:"Write Path.vi"("error in (no error)"=w322, "Path"=w314, "Configuration in"=w308) -> ("error out"=w321:errorcluster, "Configuration out"=w323:refnum<class "Configuration.lvclass">)  [unwired: 7 in]
        n134 = call <userlib>:"Read Configuration.vi"("INI Fomatted Cluster Type"=w309, "error in (no error)"=w321, "Configuration in"=w323) -> ("error out"=w319:errorcluster, "Configuration"=w320:variant, "Configuration out"=w316:refnum<class "Configuration.lvclass">)  [unwired: 6 in]
        n135 = Variant To Data(error in=w319, type=w309, Variant=w320) -> (data=w313:T15, error out=w318:errorcluster)
        n136 = Bundle By Name(cluster=w310, "Configuration"=w316, "INI"=w313) -> (w317:T16)
        n137 = call <vilib>:"Add State(s) to Queue__jki_lib_state_machine.vi"("State(s) in (\"\")"=w325) -> ("States Out"=w324:string)  [unwired: 14 in]
      }
      frame "Data: Write INI" {
        # "Do not put any code in this frame.\n(It is a separator no-op. You can make a copy of this frame to create a new Data frame)"
        n138 = local read "fake point 2"() -> (w332:dbl)
        n139 = local read "Open DAT Path"() -> (w346:path)
        n140 = local read "Export ITX Path"() -> (w345:path)
        n141 = local read "Export ITX Name"() -> (w344:string)
        n142 = local read "Intensity 1"() -> (w343:T6)
        n143 = local read "X Offset 1"() -> (w342:dbl)
        n144 = local read "derivative bin size 1"() -> (w341:dbl)
        n145 = local read "e^2/h? 1"() -> (w340:bool)
        n146 = local read "Log scale? 1"() -> (w339:bool)
        n147 = local read "fake point 1"() -> (w338:dbl)
        n148 = local read "Intensity 2"() -> (w337:T6)
        n149 = local read "X Offset 2"() -> (w336:dbl)
        n150 = local read "derivative bin size 2"() -> (w335:dbl)
        n151 = local read "e^2/h? 2"() -> (w334:bool)
        n152 = local read "Log scale? 2"() -> (w333:bool)
        n153 = Unbundle By Name(w331) -> ("Configuration"=w330:refnum<class "Configuration.lvclass">, "INI"=w326:T15)
        n154 = Bundle By Name(cluster=w326, "Open DAT Path"=w346, "Export ITX Path"=w345, "Export ITX Name"=w344, "Intensity 1"=w343, "X Offset 1"=w342, "derivative bin size 1"=w341, "e^2/h? 1"=w340, "Log scale? 1"=w339, "fake point 1"=w338, "Intensity 2"=w337, "X Offset 2"=w336, "derivative bin size 2"=w335, "e^2/h? 2"=w334, "Log scale? 2"=w333, "fake point 2"=w332) -> (w329:T15)
        n155 = call <userlib>:"Write Configuration.vi"("error in (no error)"=w328, "Variant"=w329, "Configuration in"=w330) -> ("error out"=w327:errorcluster)  [unwired: 7 in, 1 out]
        n156 = call <vilib>:"Add State(s) to Queue__jki_lib_state_machine.vi"("State(s) in (\"\")"=w348) -> ("States Out"=w347:string)  [unwired: 14 in]
      }
      frame "---------- Graph ----------" {
        # "Do not put any code in this frame.\n(It is a separator no-op. You can make a copy of this frame to create a new Data frame)"
        n157 = call <vilib>:"Add State(s) to Queue__jki_lib_state_machine.vi"("State(s) in (\"\")"=w352) -> ("States Out"=w351:string)  [unwired: 14 in]
      }
      frame "Graph: Initialize" {
        # "Do not put any code in this frame.\n(It is a separator no-op. You can make a copy of this frame to create a new Data frame)"
        n158 = control-ref of="Intensity Graph 1"() -> (w367:refnum<vi>)
        n159 = control-ref of="H Cut 1"() -> (w371:refnum<vi>)
        n160 = control-ref of="V Cut 1"() -> (w370:refnum<vi>)
        n161 = control-ref of="Intensity Graph 2"() -> (w353:refnum<vi>)
        n162 = control-ref of="H Cut 2"() -> (w368:refnum<vi>)
        n163 = control-ref of="V Cut 2"() -> (w369:refnum<vi>)
        n164 = call <userlib>:"Write Intensity Graph ref.vi"("Intensity Graph (Control)"=w353, "Intensity Graph"=w353) -> ("error out"=w356:errorcluster, "graph_utilities out"=w363:refnum<class "graph_utilities.lvclass">)  [unwired: 8 in]
        n165 = call <userlib>:"Write Intensity Graph ref.vi"("Intensity Graph (Control)"=w367, "Intensity Graph"=w367) -> ("error out"=w357:errorcluster, "graph_utilities out"=w366:refnum<class "graph_utilities.lvclass">)  [unwired: 8 in]
        n166 = call <userlib>:"Write XY Graph ref.vi"("XY Graph"=w368, "graph_utilities in"=w363) -> ("error out"=w355:errorcluster, "graph_utilities out"=w362:refnum<class "graph_utilities.lvclass">)  [unwired: 8 in]
        n167 = call <userlib>:"Write XY Graph ref.vi"("XY Graph"=w371, "graph_utilities in"=w366) -> ("error out"=w358:errorcluster, "graph_utilities out"=w365:refnum<class "graph_utilities.lvclass">)  [unwired: 8 in]
        n168 = call <userlib>:"Write XY Graph ref.vi"("XY Graph"=w369, "graph_utilities in"=w363) -> ("error out"=w354:errorcluster, "graph_utilities out"=w361:refnum<class "graph_utilities.lvclass">)  [unwired: 8 in]
        n169 = call <userlib>:"Write XY Graph ref.vi"("XY Graph"=w370, "graph_utilities in"=w366) -> ("error out"=w359:errorcluster, "graph_utilities out"=w364:refnum<class "graph_utilities.lvclass">)  [unwired: 8 in]
        n170 = Bundle By Name(cluster=w373, "Graph.Intensity 1"=w366, "Graph.H 1"=w365, "Graph.V 1"=w364, "Graph.Intensity 2"=w363, "Graph.H 2"=w362, "Graph.V 2"=w361) -> (w372:T16)
        n171 = Merge Errors(w357, w358, w359, w356, w355, w354) -> (w360:errorcluster)
        n172 = call <vilib>:"Add State(s) to Queue__jki_lib_state_machine.vi"("State(s) in (\"\")"=w375) -> ("States Out"=w374:string)  [unwired: 14 in]
      }
      frame "Graph: Set Y" {
        # "Do not put any code in this frame.\n(It is a separator no-op. You can make a copy of this frame to create a new Data frame)"
        n173 = Unbundle By Name(w390) -> ("Graph.Intensity 1"=w388:refnum<class "graph_utilities.lvclass">, "Graph.Intensity 2"=w387:refnum<class "graph_utilities.lvclass">, "Scan Names"=w386:string[], "Vfast Slice"=w377:dbl[], "Vslow Slice"=w376:dbl[])
        n174 = Index Array(array=w386) -> (element #1=w389:string, element #2=w378:string)  [unwired: 2 in]
        n175 = call <userlib>:"Set Intensity Graph Y Label.vi"("error in (no error)"=w385, "Y Label"=w389, "graph_utilities in"=w388) -> ("error out"=w383:errorcluster, "graph_utilities out"=w382:refnum<class "graph_utilities.lvclass">)  [unwired: 7 in]
        n176 = call <userlib>:"Set Intensity Graph Y Scale Array.vi"("error in (no error)"=w383, "Y Scale"=w377, "graph_utilities in"=w382) -> ("error out"=w381:errorcluster)  [unwired: 7 in, 1 out]
        n177 = call <userlib>:"Set Intensity Graph Y Label.vi"("error in (no error)"=w381, "Y Label"=w389, "graph_utilities in"=w387) -> ("error out"=w380:errorcluster, "graph_utilities out"=w384:refnum<class "graph_utilities.lvclass">)  [unwired: 7 in]
        n178 = call <userlib>:"Set Intensity Graph Y Scale Array.vi"("error in (no error)"=w380, "Y Scale"=w377, "graph_utilities in"=w384) -> ("error out"=w379:errorcluster)  [unwired: 7 in, 1 out]
        n179 = flat-sequence {
          tunnel: w378 -> [_]
          tunnel: w376 -> [_]
          frame #0 {
          }
        }
        n180 = call <vilib>:"Add State(s) to Queue__jki_lib_state_machine.vi"("State(s) in (\"\")"=w392) -> ("States Out"=w391:string)  [unwired: 14 in]
      }
      frame "Graph: Set Labels" {
        w393 = string[][] [["IV", "V_4T (V)", "I (A)"], ["IV-2T", "V_2T (V)", "I (A)"], ["d/dx(IV) R", "I (A)", "R (ohms or h/e2)"], ["d/dy(IV) G", "V_4T (V)", "G (S or e2/h)"], ["d/dx(IV-2T) R", "I (A)", "R (ohms or h/e2)"], ["d/dy(IV-2T) G", "V_2T (V)", "G (S or e2/h)"], ["d2/dy2(IV) dG/dVsg", "V_4T (V)", "dG/dVsg (e2/h/V or e2/h/meV)"], ["d2/dx2(IV) dR/dI", "I (A)", "dR/dI (h/e2/A)"]]
        # "Z scale"
        # "x scale"
        # "data"
        # "Z Scale & Label"
        # "X Scale & Label"
        # "Data Choice"
        # "Do not put any code in this frame.\n(It is a separator no-op. You can make a copy of this frame to create a new Data frame)"
        n181 = Unbundle By Name(w406) -> ("Graph.Intensity 1"=w405:refnum<class "graph_utilities.lvclass">, "Graph.Intensity 2"=w402:refnum<class "graph_utilities.lvclass">)
        n182 = Index Array(array=w393, index (row)="Intensity 1") -> (element=w401:string[])  [unwired: 1 in]
        n183 = Index Array(array=w393, index (row)="Intensity 2") -> (element=w400:string[])  [unwired: 1 in]
        n184 = Index Array(array=w401) -> (element #2=w397:string, element #3=w396:string)  [unwired: 3 in, 1 out]
        n185 = Index Array(array=w400) -> (element #2=w395:string, element #3=w394:string)  [unwired: 3 in, 1 out]
        n186 = call <userlib>:"Set Intensity Graph X Label.vi"("X Label"=w397, "graph_utilities in"=w405) -> ("graph_utilities out"=w404:refnum<class "graph_utilities.lvclass">)  [unwired: 8 in, 1 out]
        n187 = call <userlib>:"Set Intensity Graph Z Label.vi"("Z Label"=w396, "graph_utilities in"=w404) -> ()  [unwired: 8 in, 2 out]
        n188 = call <userlib>:"Set Intensity Graph X Label.vi"("X Label"=w395, "graph_utilities in"=w402) -> ("graph_utilities out"=w403:refnum<class "graph_utilities.lvclass">)  [unwired: 8 in, 1 out]
        n189 = call <userlib>:"Set Intensity Graph Z Label.vi"("Z Label"=w394, "graph_utilities in"=w403) -> ()  [unwired: 8 in, 2 out]
        n190 = call <vilib>:"Add State(s) to Queue__jki_lib_state_machine.vi"("State(s) in (\"\")"=w409) -> ("States Out"=w408:string)  [unwired: 14 in]
      }
      frame "Graph: Linecuts" {
        # "Do not put any code in this frame.\n(It is a separator no-op. You can make a copy of this frame to create a new Data frame)"
        n191 = Unbundle By Name(w420) -> ("Graph.V 1"=w419:refnum<class "graph_utilities.lvclass">, "Graph.H 1"=w416:refnum<class "graph_utilities.lvclass">, "Graph.V 2"=w417:refnum<class "graph_utilities.lvclass">, "Graph.H 2"=w418:refnum<class "graph_utilities.lvclass">)  [unwired: 2 out]
        n192 = call <userlib>:"Intensity Graph Linecut (Vertical).vi"("error in (no error)"=w411, "graph_utilities in"=w419) -> ("error out"=w415:errorcluster)  [unwired: 8 in, 1 out]
        n193 = call <userlib>:"Intensity Graph Linecut (Horizontal).vi"("error in (no error)"=w411, "graph_utilities in"=w416) -> ("error out"=w414:errorcluster)  [unwired: 8 in, 1 out]
        n194 = call <userlib>:"Intensity Graph Linecut (Vertical).vi"("error in (no error)"=w411, "graph_utilities in"=w417) -> ("error out"=w413:errorcluster)  [unwired: 8 in, 1 out]
        n195 = call <userlib>:"Intensity Graph Linecut (Horizontal).vi"("error in (no error)"=w411, "graph_utilities in"=w418) -> ("error out"=w412:errorcluster)  [unwired: 8 in, 1 out]
        n196 = Merge Errors(w415, w414, w413, w412) -> (w410:errorcluster)
        n197 = call <vilib>:"Add State(s) to Queue__jki_lib_state_machine.vi"("State(s) in (\"\")"=w422) -> ("States Out"=w421:string)  [unwired: 14 in]
      }
      frame "---------- UI ----------" {
        # "Do not put any code in this frame.\n(It is a separator no-op. You can make a copy of this frame to create a new UI frame)"
        n198 = call <vilib>:"Add State(s) to Queue__jki_lib_state_machine.vi"("State(s) in (\"\")"=w426) -> ("States Out"=w425:string)  [unwired: 14 in]
      }
      frame "UI: Initialize" {
        # "Initialize the User Interface, here.\n(this is called automatically, by the Macro: Init)"
        n199 = Unbundle By Name(w429) -> ("Core.Current VI Reference"=w428:refnum<vi>)
        n200 = property class="VI" props=["FP.Behavior"](reference=w428) -> ()  [unwired: 1 in, 3 out]
        n201 = local write "OK"(FALSE ("OK")) -> ()
        n202 = local write "Field/Temperature"(0 ("Field/Temperature")) -> ()
        n203 = local write "Tab Control"(T13."Intensity Graphs" ("Tab Control")) -> ()
        n204 = call <userlib>:"Fit VI window to Largest Dec__ogtk.vi"("error in (no error)"=w432, "border spacing (2 px)"=-2) -> ("error out"=w431:errorcluster)  [unwired: 4 in, 1 out]
        n205 = call <vilib>:"Add State(s) to Queue__jki_lib_state_machine.vi"("State(s) in (\"\")"=w436) -> ("States Out"=w435:string)  [unwired: 14 in]
      }
      frame "UI: Initialize Controls" {
        # "Do not put any code in this frame.\n(It is a separator no-op. You can make a copy of this frame to create a new UI frame)"
        n206 = Unbundle By Name(w438) -> ("INI"=w437:T15)
        n207 = Unbundle By Name(w437) -> ("Open DAT Path"=w453:path, "Export ITX Path"=w452:path, "Export ITX Name"=w451:string, "Intensity 1"=w450:T6, "X Offset 1"=w449:dbl, "derivative bin size 1"=w448:dbl, "e^2/h? 1"=w447:bool, "Log scale? 1"=w446:bool, "fake point 1"=w445:dbl, "Intensity 2"=w444:T6, "X Offset 2"=w443:dbl, "derivative bin size 2"=w442:dbl, "e^2/h? 2"=w441:bool, "Log scale? 2"=w440:bool, "fake point 2"=w439:dbl)
        n208 = local write "fake point 2"(w439) -> ()
        n209 = local write "Open DAT Path"(w453) -> ()
        n210 = local write "Export ITX Path"(w452) -> ()
        n211 = local write "Export ITX Name"(w451) -> ()
        n212 = local write "Intensity 1"(w450) -> ()
        n213 = local write "X Offset 1"(w449) -> ()
        n214 = local write "derivative bin size 1"(w448) -> ()
        n215 = local write "e^2/h? 1"(w447) -> ()
        n216 = local write "Log scale? 1"(w446) -> ()
        n217 = local write "fake point 1"(w445) -> ()
        n218 = local write "Intensity 2"(w444) -> ()
        n219 = local write "X Offset 2"(w443) -> ()
        n220 = local write "derivative bin size 2"(w442) -> ()
        n221 = local write "e^2/h? 2"(w441) -> ()
        n222 = local write "Log scale? 2"(w440) -> ()
        n223 = call <vilib>:"Add State(s) to Queue__jki_lib_state_machine.vi"("State(s) in (\"\")"=w456) -> ("States Out"=w455:string)  [unwired: 14 in]
      }
      frame "UI: Cursor Set" {
        # "Argument"
        # "Set and Unset Cursor Busy.\n(Usage: \"UI: Cursor Set >> Busy|Idle\")"
        n224 = case shown="\"Idle\", Default" w457 {
          tunnel: w459 -> [w464 w466]
          tunnel: [w463 w465] -> w458
          frame "Idle", Default {
            n225 = call <vilib>:"Unset Busy.vi"("error in (no error)"=w464) -> ("error out"=w463:errorcluster)  [unwired: 10 in]
          }
          frame "Busy" {
            n226 = call <vilib>:"Set Busy.vi"("error in (no error)"=w466) -> ("error out"=w465:errorcluster)  [unwired: 9 in, 1 out]
          }
        }
        n227 = call <vilib>:"Add State(s) to Queue__jki_lib_state_machine.vi"("State(s) in (\"\")"=w462) -> ("States Out"=w461:string)  [unwired: 14 in]
      }
      frame "UI: Front Panel State" {
        # "Argument"
        # "Set Front Panel Open or Closed\n(Usage: \"UI: Front Panel State >> Open|Close\")"
        n228 = Unbundle By Name(w469) -> ("Core.Current VI Reference"=w468:refnum<vi>)
        n229 = case shown="\"Minimize\", \"Minimized\"" w467 {
          tunnel: w471 -> [w479 w494 w505 w518 w531]
          tunnel: [w481 w495 w507 w520 w533] -> w470
          tunnel: w468 -> [w480 w492 w506 w519 w532]
          frame "Open", "Standard", Default {
            w474 = T11."Standard" ("State")
            n230 = property class="VI"(reference=w480, error in=w479) -> (reference out=w477:refnum<vi>, error out=w478:errorcluster, "FP.State"=w476:T11)
            n231 = Not Equal?(x=w476, y=w474) -> (x != y?=w475:bool)
            n232 = case shown="True" w475 {
              tunnel: [w485 w487] -> w481
              tunnel: w478 -> [w484 w487]
              tunnel: w477 -> [w483 _]
              tunnel: w474 -> [w482 _]
              frame True {
                n233 = invoke class="VI" method="FP.Open"(reference=w483, error in=w484, "Activate"=TRUE, "State"=w482) -> (error out=w485:errorcluster)  [unwired: 1 in, 4 out]
              }
              frame False {
              }
            }
          }
          frame "Close", "Closed" {
            n234 = property class="VI"(reference=w492, error in=w494) -> (reference out=w491:refnum<vi>, error out=w493:errorcluster, "FP.State"=w489:T11)
            n235 = Not Equal?(x=w489, y=T11."Closed" ("Front Panel Window:State")) -> (x != y?=w488:bool)
            n236 = case shown="True" w488 {
              tunnel: [w496 w499] -> w495
              tunnel: w493 -> [w496 w498]
              tunnel: w491 -> [_ w497]
              frame False {
              }
              frame True {
                n237 = invoke class="VI" method="FP.Close"(reference=w497, error in=w498) -> (error out=w499:errorcluster)  [unwired: 1 in, 2 out]
              }
            }
          }
          frame "Hidden", "Hide" {
            w500 = T11."Hidden" ("State")
            n238 = property class="VI"(reference=w506, error in=w505) -> (reference out=w503:refnum<vi>, error out=w504:errorcluster, "FP.State"=w502:T11)
            n239 = Not Equal?(x=w502, y=w500) -> (x != y?=w501:bool)
            n240 = case shown="True" w501 {
              tunnel: [w511 w512] -> w507
              tunnel: w504 -> [w510 w512]
              tunnel: w503 -> [w509 _]
              tunnel: w500 -> [w508 _]
              frame True {
                n241 = invoke class="VI" method="FP.Open"(reference=w509, error in=w510, "State"=w508) -> (error out=w511:errorcluster)  [unwired: 2 in, 4 out]
              }
              frame False {
              }
            }
          }
          frame "Minimize", "Minimized" {
            w513 = T11."Minimized" ("State")
            n242 = property class="VI"(reference=w519, error in=w518) -> (reference out=w516:refnum<vi>, error out=w517:errorcluster, "FP.State"=w515:T11)
            n243 = Not Equal?(x=w515, y=w513) -> (x != y?=w514:bool)
            n244 = case shown="True" w514 {
              tunnel: [w524 w525] -> w520
              tunnel: w517 -> [w523 w525]
              tunnel: w516 -> [w522 _]
              tunnel: w513 -> [w521 _]
              frame True {
                n245 = invoke class="VI" method="FP.Open"(reference=w522, error in=w523, "State"=w521) -> (error out=w524:errorcluster)  [unwired: 2 in, 4 out]
              }
              frame False {
              }
            }
          }
          frame "Maximize", "Maximized" {
            w526 = T11."Maximized" ("State")
            n246 = property class="VI"(reference=w532, error in=w531) -> (reference out=w529:refnum<vi>, error out=w530:errorcluster, "FP.State"=w528:T11)
            n247 = Not Equal?(x=w528, y=w526) -> (x != y?=w527:bool)
            n248 = case shown="True" w527 {
              tunnel: [w537 w538] -> w533
              tunnel: w530 -> [w536 w538]
              tunnel: w529 -> [w535 _]
              tunnel: w526 -> [w534 _]
              frame True {
                n249 = invoke class="VI" method="FP.Open"(reference=w535, error in=w536, "State"=w534) -> (error out=w537:errorcluster)  [unwired: 2 in, 4 out]
              }
              frame False {
              }
            }
          }
        }
        n250 = call <vilib>:"Add State(s) to Queue__jki_lib_state_machine.vi"("State(s) in (\"\")"=w473) -> ("States Out"=w472:string)  [unwired: 14 in]
      }
      frame "UI: Choose Tab" {
        # "Do not put any code in this frame.\n(It is a separator no-op. You can make a copy of this frame to create a new UI frame)"
        n251 = case shown="\"Intensity Graphs\", Default" w540 {
          tunnel: [T13."Intensity Graphs" ("Value (Signaling)")] -> w539
          frame "Intensity Graphs", Default {
          }
        }
        n252 = disable-structure shown="Disabled" {
          frame Disabled {
            n253 = property on="Tab Control" class="TabCtl (strict)"() -> ("Pages"=w545:refnum<vi>[])  [unwired: 2 in, 2 out]
            n254 = for {
              tunnel: w545 -> [w547] mode=indexing
              tunnel: [w546] -> _ mode=indexing
              n255 = property class="Page"(reference=w547) -> ("PageLabel"=w546:string)  [unwired: 1 in, 2 out]
            }
          }
          frame Enabled {
          }
        }
        n256 = property on="Tab Control" class="TabCtl (strict)"("Val(Sgnl)"=w539) -> ()  [unwired: 2 in, 2 out]
        n257 = call <vilib>:"Add State(s) to Queue__jki_lib_state_machine.vi"("State(s) in (\"\")"=w544) -> ("States Out"=w543:string)  [unwired: 14 in]
      }
      frame "---------- Macro ----------" {
        # "Do not put any code in this frame.\n(It is a separator no-op. You can make a copy of this frame to create a new Macro frame)"
        n258 = call <vilib>:"Add State(s) to Queue__jki_lib_state_machine.vi"("State(s) in (\"\")"=w552) -> ("States Out"=w551:string)  [unwired: 14 in]
      }
      frame "Macro: Initialize" {
        # "Initialization Macro\n(This is called once, when the VI starts)"
        n259 = call <vilib>:"Add State(s) to Queue__jki_lib_state_machine.vi"("State(s) in Front (\"\")"="Data: Initialize\nInitialize Core Data\nUI: Initialize\nUI: Front Panel State >> Open\n\nData: Read INI\nUI: Initialize Controls\n\nGraph: Initialize\nData Visualize: Initialize DVRs", "State(s) in (\"\")"=w557) -> ("States Out"=w556:string)  [unwired: 13 in]
      }
      frame "Macro: Exit" {
        # "Exit Macro\n(This is called once, when the VI exits)"
        n260 = Unbundle By Name(w565) -> ("Core.Close Panel on Exit?"=w564:bool)
        n261 = Select(t="UI: Front Panel State >> Close", s=w564, f="") -> (s? t:f=w561:string)
        n262 = call <vilib>:"Add State(s) to Queue__jki_lib_state_machine.vi"("State(s) in Front (\"\")"="Data: Write INI\nData Visualize: Cleanup DVRs", "State(s) in (\"\")"=w561, "State(s) at Back (\"\")"="Data: Cleanup\nExit") -> ("States Out"=w559:string)  [unwired: 12 in]
        n263 = call <vilib>:"Add State(s) to Queue__jki_lib_state_machine.vi"("State(s) in Front (\"\")"=w559, "State(s) in (\"\")"=w568) -> ("States Out"=w567:string)  [unwired: 13 in]
      }
      frame "Macro: Update Graphs" {
        # "Do not put any code in this frame.\n(It is a separator no-op. You can make a copy of this frame to create a new Macro frame)"
        n264 = call <vilib>:"Add State(s) to Queue__jki_lib_state_machine.vi"("State(s) in (\"\")"=w572) -> ("States Out"=w571:string)  [unwired: 14 in]
      }
      frame "Macro: Visualize" {
        # "Do not put any code in this frame.\n(It is a separator no-op. You can make a copy of this frame to create a new Macro frame)"
        n265 = call <vilib>:"Add State(s) to Queue__jki_lib_state_machine.vi"("State(s) in Front (\"\")"="Data Visualize: Read DAT File\nData Visualize: Cleanup DVRs\nData Visualize: Initialize DVRs\nData Visualize: Initialize Cursor Graph\nData Visualize: Subset\nData Visualize: Testing\nData Visualize: SG Filter\nData Visualize: Calculate Derivative\n\nData Visualize: Calculate Indices\nGraph: Initialize\nGraph: Set Y\nGraph: Set Labels\n//Data Visualize: Calculate Indices\n//Data Visualize: Choose Data 1\n//Data Visualize: Choose Data 2\n//Graph: Linecuts\nUI: Choose Tab >> Intensity Graphs\nUI: Cursor Set >> Idle" ("State(s) in Front (\"\")"), "State(s) in (\"\")"=w577) -> ("States Out"=w576:string)  [unwired: 13 in]
      }
      frame "Macro: Generate" {
        # "Do not put any code in this frame.\n(It is a separator no-op. You can make a copy of this frame to create a new Macro frame)"
        n266 = call <vilib>:"Add State(s) to Queue__jki_lib_state_machine.vi"("State(s) in Front (\"\")"="Data Generation: Update Class Wire\nData Generation: Read ITX Files\nData Generation: Write DAT File" ("State(s) in Front (\"\")"), "State(s) in (\"\")"=w582) -> ("States Out"=w581:string)  [unwired: 13 in]
      }
      frame "---------- Data Generation ----------" {
        # "Template Separator\n(You can make a copy of, or modify, this frame)"
        n267 = call <vilib>:"Add State(s) to Queue__jki_lib_state_machine.vi"("State(s) in (\"\")"=w586) -> ("States Out"=w585:string)  [unwired: 14 in]
      }
      frame "Data Generation: Update Class Wire" {
        # "Template Separator\n(You can make a copy of, or modify, this frame)"
        n268 = Unbundle By Name(w594) -> ("Retrieve and Visualize"=w596:refnum<class "Retrieve and Visualize.lvclass">)
        n269 = Bundle By Name(cluster=w596, "File or Folder Path"="Path", "T/B third axis"="T/B third axis", "IV setup"="IV setup", "index"=T14 {"V2T"="", "V+"="", "V-"="", "I (A)"="", "+X"="", "+Y"="", "-X"="", "-Y"="", "B"=""} ("Data Generation.index"), "Portion of data"="Portion of data (%)", "Decimate point"="Decimate point", "Parameters from comments?"="Extract paramaters from comments?", "Scan names"="Scan names") -> (w595:refnum<class "Retrieve and Visualize.lvclass">)
        n270 = Bundle By Name(cluster=w594, "Retrieve and Visualize"=w595) -> (w593:T16)
        n271 = call <vilib>:"Add State(s) to Queue__jki_lib_state_machine.vi"("State(s) in (\"\")"=w601) -> ("States Out"=w600:string)  [unwired: 14 in]
      }
      frame "Data Generation: Read ITX Files" {
        # "Your code here.\n(You can make a copy of, or modify, this frame)"
        n272 = Unbundle By Name(w607) -> ("Retrieve and Visualize"=w608:refnum<class "Retrieve and Visualize.lvclass">)
        n273 = for {
          N: "# of fields/Temperatures" -> [w616]
          shift-right: [w623] -> w605
          shift-left: w608 -> [w620]
          tunnel: [w613] -> w603
          tunnel: w604 -> [w612]
          i -> [w615]
          n274 = Multiply(x=w615, y="Field Period") -> (x*y=w619:i32)
          n275 = Bundle By Name(cluster=w620, "# of B/T"=w616, "B/T offset"=w619, "Field Period"="Field Period") -> (w617:refnum<class "Retrieve and Visualize.lvclass">)
          n276 = call "Data retrieve engine_SE.vi"("error in (no error)"=w612, "File Type"="File Type", "Retrieve and Visualize"=w617) -> ("error out"=w622:errorcluster, "Retrieve and Visualize out"=w621:refnum<class "Retrieve and Visualize.lvclass">)  [unwired: 7 in]
          n277 = call "Create DAT Comments.vi"("error in"=w622, "Additional comments"="Additional comments", "Retrieve and Visualize"=w621) -> ("error out"=w613:errorcluster, "Retrieve and Visualize out"=w623:refnum<class "Retrieve and Visualize.lvclass">)  [unwired: 7 in]
        }
        n278 = Bundle By Name(cluster=w607, "Retrieve and Visualize"=w605) -> (w606:T16)
        n279 = call <vilib>:"Add State(s) to Queue__jki_lib_state_machine.vi"("State(s) in (\"\")"=w610) -> ("States Out"=w609:string)  [unwired: 14 in]
      }
      frame "Data Generation: Check Files" {
        # "Template Separator\n(You can make a copy of, or modify, this frame)"
        n280 = disable-structure shown="Disabled" {
          frame Disabled {
            n281 = local read "Path"() -> (w632:path)
            n282 = local read "index"() -> ()  [unwired: 1 out]
            n283 = local read "File Type"() -> (w631:T5)
            n284 = call "LV to ITX Retrieve_SE mode_aditi.vi"("File or Folder Path"=w632, "offset"=0, "length"=1, "stop"=FALSE, "File Type"=w631) -> ()  [unwired: 4 in, 7 out]
          }
          frame Enabled {
          }
        }
        n285 = call <vilib>:"Add State(s) to Queue__jki_lib_state_machine.vi"("State(s) in (\"\")"=w627) -> ("States Out"=w626:string)  [unwired: 14 in]
      }
      frame "Data Generation: Write DAT File" {
        # "Your code here.\n(You can make a copy of, or modify, this frame)"
        n286 = Unbundle By Name(w636) -> ("Retrieve and Visualize"=w635:refnum<class "Retrieve and Visualize.lvclass">)
        n287 = call "Create DAT File.vi"("error in"=w638, "DAT file name"="IV file name", "Processed data folder"="DAT folder", "Retrieve and Visualize"=w635) -> ("error out"=w637:errorcluster)  [unwired: 6 in, 1 out]
        n288 = call <vilib>:"Add State(s) to Queue__jki_lib_state_machine.vi"("State(s) in (\"\")"=w640) -> ("States Out"=w639:string)  [unwired: 14 in]
      }
      frame "---------- Data Visualize ----------" {
        # "Template Separator\n(You can make a copy of, or modify, this frame)"
        n289 = call <vilib>:"Add State(s) to Queue__jki_lib_state_machine.vi"("State(s) in (\"\")"=w644) -> ("States Out"=w643:string)  [unwired: 14 in]
      }
      frame "Data Visualize: Read DAT File" {
        # "Template Separator\n(You can make a copy of, or modify, this frame)"
        n290 = Empty String/Path?(string/path="Open DAT Path") -> (empty?=w650:bool)
        n291 = call-poly <userlib>:"File Exists__ogtk.vi"("file path"="Open DAT Path") -> ("exists"=w652:bool)  [unwired: 6 in, 1 out]
        n292 = Not(x=w652) -> (.not. x?=w651:bool)
        n293 = Or(x=w650, y=w651) -> ()  [unwired: 1 out]
        n294 = call <vilib>:"Get File Extension.vi"("error in (no error)"=w646, "file"="Open DAT Path") -> ("error out"=w645:errorcluster, "lowercase file extension"=w649:string, "dup file"=w647:path)  [unwired: 5 in, 2 out]
        n295 = case shown="Default" w649 {
          tunnel: [w662 w665] -> w653
          tunnel: w647 -> [w662 _]
          tunnel: w645 -> [w661 w667]
          tunnel: [w661 w666] -> w654
          frame "dat" {
          }
          frame Default {
            w663 = "DAT" ("pattern label")
            n296 = call "File Dialog"("button label"=w663, "error in"=w667, "pattern (all files)"="*.dat", "pattern label"=w663) -> ("selected path"=w665:path, "error out"=w666:errorcluster)  [unwired: 8 in, 2 out]
          }
        }
        n297 = call "Read DAT File.vi"("error in"=w654, "file path (use dialog)"=w653) -> ("error out"=w658:errorcluster, "Retrieve and Visualize out"=w657:refnum<class "Retrieve and Visualize.lvclass">)  [unwired: 8 in]
        n298 = local write "Open DAT Path"(w653) -> ()
        n299 = Bundle By Name(cluster=w656, "Retrieve and Visualize"=w657) -> (w655:T16)
        n300 = call <vilib>:"Add State(s) to Queue__jki_lib_state_machine.vi"("State(s) in (\"\")"=w660) -> ("States Out"=w659:string)  [unwired: 14 in]
      }
      frame "Data Visualize: Initialize DVRs" {
        w669 = cluster{dbl[], dbl[]}[][][] [] ("DAT File.IV-2T")
        # "Template Separator\n(You can make a copy of, or modify, this frame)"
        n301 = Unbundle By Name(w689) -> ("Retrieve and Visualize"=w690:refnum<class "Retrieve and Visualize.lvclass">)
        n302 = Unbundle By Name(w690) -> ("IV"=w691:cluster{dbl[], dbl[]}[][][], "IV-2T"=w675:cluster{dbl[], dbl[]}[][][], "Vfast"=w685:dbl[][], "Vslow"=w684:dbl[], "Vslowest"=w683:dbl[], "Comments"=→"Comments":string, "Scan names"=w668:string[])
        n303 = New Data Value Reference(data value=w691, error in=w682) -> (data value reference=w687:refnum<data-value>, error out=w680:errorcluster)
        n304 = New Data Value Reference(data value=w675, error in=w680) -> (data value reference=w686:refnum<data-value>, error out=w679:errorcluster)
        n305 = New Data Value Reference(data value=w669, error in=w679) -> (data value reference=w671:refnum<data-value>, error out=w678:errorcluster)
        n306 = New Data Value Reference(data value=w669, error in=w678) -> (data value reference=w672:refnum<data-value>, error out=w677:errorcluster)
        n307 = New Data Value Reference(data value=w669, error in=w677) -> (data value reference=w673:refnum<data-value>, error out=w676:errorcluster)
        n308 = New Data Value Reference(data value=w669, error in=w676) -> (data value reference=w674:refnum<data-value>, error out=w681:errorcluster)
        n309 = Bundle By Name(cluster=w689, "DVR.IV-4T"=w687, "DVR.IV-2T"=w686, "DVR.G-4T"=w671, "DVR.R-4T"=w672, "DVR.G-2T"=w673, "DVR.R-2T"=w674, "Vfast"=w685, "Vslow"=w684, "Vslowest"=w683, "Scan Names"=w668) -> (w688:T16)
        n310 = call <vilib>:"Add State(s) to Queue__jki_lib_state_machine.vi"("State(s) in (\"\")"=w693) -> ("States Out"=w692:string)  [unwired: 14 in]
      }
      frame "Data Visualize: Cleanup DVRs" {
        # "Template Separator\n(You can make a copy of, or modify, this frame)"
        n311 = Unbundle By Name(w698) -> ("DVR"=w697:T18)
        n312 = Unbundle By Name(w697) -> ("IV-4T"=w695:refnum<data-value>, "G-2T"=w709:refnum<data-value>, "R-2T"=w708:refnum<data-value>, "G-4T"=w707:refnum<data-value>, "R-4T"=w706:refnum<data-value>, "IV-2T"=w705:refnum<data-value>)
        n313 = Delete Data Value Reference(data value reference=w705) -> (error out=w704:errorcluster)  [unwired: 1 in, 1 out]
        n314 = Delete Data Value Reference(data value reference=w706) -> (error out=w699:errorcluster)  [unwired: 1 in, 1 out]
        n315 = Delete Data Value Reference(data value reference=w707) -> (error out=w700:errorcluster)  [unwired: 1 in, 1 out]
        n316 = Delete Data Value Reference(data value reference=w708) -> (error out=w701:errorcluster)  [unwired: 1 in, 1 out]
        n317 = Delete Data Value Reference(data value reference=w709) -> (error out=w702:errorcluster)  [unwired: 1 in, 1 out]
        n318 = Delete Data Value Reference(data value reference=w695) -> (error out=w703:errorcluster)  [unwired: 1 in, 1 out]
        n319 = Merge Errors(w703, w702, w701, w700, w699, w704) -> (w694:errorcluster)
        n320 = disable-structure shown="Enabled" {
          disable-tunnel: w694 -> [w712 _]
          frame Disabled {
            n321 = flat-sequence {
              tunnel: w712 -> [_]
              frame #0 {
                n322 = Request Deallocation(TRUE ("flag")) -> ()
              }
            }
          }
          frame Enabled {
          }
        }
        n323 = call <vilib>:"Clear Errors.vi"("error in (no error)"=w694) -> ("error out"=w696:errorcluster)  [unwired: 5 in, 1 out]
        n324 = call <vilib>:"Add State(s) to Queue__jki_lib_state_machine.vi"("State(s) in (\"\")"=w711) -> ("States Out"=w710:string)  [unwired: 14 in]
      }
      frame "Data Visualize: Initialize Cursor Graph" {
        w718 = dbl[] []
        # "Initialize Cursor Graph"
        # "replace with array resize?"
        # "Do not put any code in this frame.\n(It is a separator no-op. You can make a copy of this frame to create a new UI frame)"
        n325 = Unbundle By Name(w714) -> ("Vfast"=w720:dbl[][], "Vslow"=w719:dbl[], "Scan Names"=w724:string[])
        n326 = Transpose 2D Array(2D array=w720) -> (transposed array=w715:dbl[][])
        n327 = for {
          tunnel: w715 -> [w733] mode=indexing
          tunnel: w719 -> [w730]
          shift-right: [w731] -> w721
          shift-left: w718 -> [w732]
          shift-right: [w729] -> w722
          shift-left: w718 -> [w728]
          n328 = Build Array (concatenate)(w732, w733) -> (w731:dbl[])
          n329 = Build Array (concatenate)(w728, w730) -> (w729:dbl[])
        }
        n330 = Index Array(array=w724) -> (element #1=w716:string, element #2=w723:string)  [unwired: 2 in]
        n331 = property on="Cursor Graph" class="XYGraph (strict)"("XScale.NameLbl.Text"=w716, "YScale.NameLbl.Text"=w723) -> ()  [unwired: 2 in, 2 out]
        n332 = Bundle(w721, w722) -> (→"Cursor Graph":cluster{dbl[], dbl[]})  [unwired: 1 in]
        n333 = call <vilib>:"Add State(s) to Queue__jki_lib_state_machine.vi"("State(s) in (\"\")"=w727) -> ("States Out"=w726:string)  [unwired: 14 in]
      }
      frame "Data Visualize: Calculate Derivative" {
        w747 = enum16{"y/x vs x", "x/y vs y"}."y/x vs x" ("Type 2")
        w748 = enum16{"y/x vs x", "x/y vs y"}."x/y vs y" ("Type 2")
        # "Template Separator\n(You can make a copy of, or modify, this frame)"
        n334 = Unbundle By Name(w755) -> ("DVR.IV-4T"=w742:refnum<data-value>, "DVR.G-4T"=w746:refnum<data-value>, "DVR.R-4T"=w745:refnum<data-value>, "DVR.IV-2T"=w741:refnum<data-value>, "DVR.G-2T"=w744:refnum<data-value>, "DVR.R-2T"=w743:refnum<data-value>)
        n335 = call "Derivative (DVR).vi"("Type"=w748, "Data Value Reference in"=w742, "error in (no error)"=w749, "Interval Units (points)"="Interval Units (points)", "Window [h] (2)"="Window [h] (2)", "dX in"=w746) -> ("error out"=w737:errorcluster, "dX out"=w750:refnum<data-value>)  [unwired: 4 in]
        n336 = call "Derivative (DVR).vi"("Type"=w747, "Data Value Reference in"=w742, "Interval Units (points)"="Interval Units (points)", "Window [h] (2)"="Window [h] (2)", "dX in"=w745) -> ("error out"=w738:errorcluster, "dX out"=w751:refnum<data-value>)  [unwired: 5 in]
        n337 = call "Derivative (DVR).vi"("Type"=w748, "Data Value Reference in"=w741, "Interval Units (points)"="Interval Units (points)", "Window [h] (2)"="Window [h] (2)", "dX in"=w744) -> ("error out"=w739:errorcluster, "dX out"=w752:refnum<data-value>)  [unwired: 5 in]
        n338 = call "Derivative (DVR).vi"("Type"=w747, "Data Value Reference in"=w741, "Interval Units (points)"="Interval Units (points)", "Window [h] (2)"="Window [h] (2)", "dX in"=w743) -> ("error out"=w740:errorcluster, "dX out"=w753:refnum<data-value>)  [unwired: 5 in]
        n339 = Bundle By Name(cluster=w755, "DVR.G-4T"=w750, "DVR.R-4T"=w751, "DVR.G-2T"=w752, "DVR.R-2T"=w753) -> (w754:T16)
        n340 = Merge Errors(w740, w739, w738, w737) -> (w736:errorcluster)
        n341 = call <vilib>:"Add State(s) to Queue__jki_lib_state_machine.vi"("State(s) in (\"\")"=w757) -> ("States Out"=w756:string)  [unwired: 14 in]
      }
      frame "Data Visualize: SG Filter" {
        # "Template Separator\n(You can make a copy of, or modify, this frame)"
        n342 = Unbundle By Name(w767) -> ("DVR.IV-4T"=w769:refnum<data-value>, "DVR.IV-2T"=w759:refnum<data-value>)
        n343 = call "SG Filter (DVR).vi"("error in"=w764, "side points"="S-G side points (4T)", "Data Value Reference in"=w769) -> ("error out"=w761:errorcluster, "Data Value Reference out"=w768:refnum<data-value>)  [unwired: 7 in]
        n344 = call "SG Filter (DVR).vi"("side points"="S-G side points (2T)", "Data Value Reference in"=w759) -> ("error out"=w762:errorcluster, "Data Value Reference out"=w765:refnum<data-value>)  [unwired: 8 in]
        n345 = disable-structure shown="Enabled" {
          disable-tunnel: _ -> [w777 _]
          disable-tunnel: _ -> [w776 _]
          disable-tunnel: w762 -> [w775 w778]
          disable-tunnel: [w773 w778] -> _
          disable-tunnel: _ -> [w772 _]
          frame Disabled {
            n346 = call "SG Filter (DVR).vi"("error in"=w775, "side points"=w772, "Data Value Reference in"=w777) -> ("error out"=w774:errorcluster)  [unwired: 7 in, 1 out]
            n347 = call "SG Filter (DVR).vi"("error in"=w774, "side points"=w772, "Data Value Reference in"=w776) -> ("error out"=w773:errorcluster)  [unwired: 7 in, 1 out]
          }
          frame Enabled {
          }
        }
        n348 = Merge Errors(w762, w761) -> (w760:errorcluster)
        n349 = Bundle By Name(cluster=w767, "DVR.IV-4T"=w768, "DVR.IV-2T"=w765) -> (w766:T16)
        n350 = call <vilib>:"Add State(s) to Queue__jki_lib_state_machine.vi"("State(s) in (\"\")"=w771) -> ("States Out"=w770:string)  [unwired: 14 in]
      }
      frame "Data Visualize: Subset" {
        # "Template Separator\n(You can make a copy of, or modify, this frame)"
        n351 = Unbundle By Name(w789) -> ("DVR.IV-4T"=w786:refnum<data-value>, "DVR.IV-2T"=w784:refnum<data-value>)
        n352 = call "Subset (DVR).vi"("error in"=w780, "Subset Slider (%)"="Subset Slider (%)", "Data Value Reference in"=w786) -> ("error out"=w781:errorcluster, "Data Value Reference out"=w785:refnum<data-value>)  [unwired: 7 in]
        n353 = call "Subset (DVR).vi"("error in"=w780, "Subset Slider (%)"="Subset Slider (%)", "Data Value Reference in"=w784) -> ("error out"=w782:errorcluster, "Data Value Reference out"=w779:refnum<data-value>)  [unwired: 7 in]
        n354 = Merge Errors(w782, w781) -> (w787:errorcluster)
        n355 = Bundle By Name(cluster=w789, "DVR.IV-4T"=w785, "DVR.IV-2T"=w779) -> (w788:T16)
        n356 = call <vilib>:"Add State(s) to Queue__jki_lib_state_machine.vi"("State(s) in (\"\")"=w791) -> ("States Out"=w790:string)  [unwired: 14 in]
      }
      frame "Data Visualize: Testing" {
        # "Template Separator\n(You can make a copy of, or modify, this frame)"
        n357 = Unbundle By Name(w801) -> ("DVR.IV-4T"=w798:refnum<data-value>, "DVR.IV-2T"=w796:refnum<data-value>)
        n358 = call "Testing (DVR).vi"("error in"=w794, "Data Value Reference in"=w798) -> ("error out"=w793:errorcluster, "Data Value Reference out"=w797:refnum<data-value>)  [unwired: 8 in]
        n359 = call "Testing (DVR).vi"("error in"=w794, "Data Value Reference in"=w796) -> ("error out"=w792:errorcluster, "Data Value Reference out"=w795:refnum<data-value>)  [unwired: 8 in]
        n360 = Merge Errors(w792, w793) -> (w799:errorcluster)
        n361 = Bundle By Name(cluster=w801, "DVR.IV-4T"=w797, "DVR.IV-2T"=w795) -> (w800:T16)
        n362 = call <vilib>:"Add State(s) to Queue__jki_lib_state_machine.vi"("State(s) in (\"\")"=w803) -> ("States Out"=w802:string)  [unwired: 14 in]
      }
      frame "Data Visualize: Calculate Indices" {
        # "used?"
        # "used?"
        # "used?"
        # "used?"
        # "Calculate Indices"
        # "Template Separator\n(You can make a copy of, or modify, this frame)"
        n363 = Unbundle By Name(w814) -> ("Vfast"=w817:dbl[][], "Vslow"=w816:dbl[], "Vslowest"=w815:dbl[])
        n364 = property on="Cursor Graph" class="XYGraph (strict)"(error in=w805) -> (error out=w804:errorcluster, "Cursor.Cursor X"=w823:dbl, "Cursor.Cursor Y"=w822:dbl)  [unwired: 1 in, 1 out]
        "Slow" <- w822
        "Fast" <- w823
        n365 = local read "Field/Temperature"() -> (w820:i32)
        n366 = Index Array(array=w815, index=w820) -> (element=→"slowest":dbl)
        n367 = call "Calculate Indices.vi"("Cursor.Cursor Y"=w822, "Cursor.Cursor X"=w823, "Vslow"=w816, "Vfast"=w817) -> ("Column"=w806:i32, "Row"=w807:i32, "Column Array"=w808:i32[], "Row Array"=w809:i32[])  [unwired: 4 in]
        n368 = Array Size(array=w815) -> (size(s)=w818:i32)
        n369 = Decrement(x=w818) -> (x-1=w819:i32)
        n370 = Index Array(array=w817, index (row)=w807) -> (element=w811:dbl[])  [unwired: 1 in]
        n371 = property on="Field/Temperature" class="Slide (strict)"("Scale.Maximum"=w819) -> ()  [unwired: 2 in, 2 out]
        n372 = Reverse 1D Array(array=w816) -> (reversed array=w812:dbl[])
        n373 = Bundle By Name(cluster=w814, "Vfast Slice"=w811, "Vslow Slice"=w812, "Page"="Field/Temperature", "Row Array"=w809, "Column Array"=w808, "Row"=w807, "Column"=w806) -> (w813:T16)
        n374 = call <vilib>:"Add State(s) to Queue__jki_lib_state_machine.vi"("State(s) in (\"\")"=w825) -> ("States Out"=w824:string)  [unwired: 14 in]
      }
      frame "Data Visualize: Vary Vfast" {
        # "Template Separator\n(You can make a copy of, or modify, this frame)"
        n375 = Unbundle By Name(w828) -> ("DVR.IV-4T"=w829:refnum<data-value>, "DVR.G-2T"=w834:refnum<data-value>, "DVR.R-2T"=w830:refnum<data-value>, "DVR.G-4T"=w831:refnum<data-value>, "DVR.R-4T"=w832:refnum<data-value>, "DVR.IV-2T"=w833:refnum<data-value>, "Page"=w826:i32, "Row"=w827:i32)
        n376 = in-place {
          in-place-border: w826 -> [w846]
          in-place-border: w827 -> [w844]
          n377 = in-place-dvr #3(w829) -> (w843:cluster{dbl[], dbl[]}[][][])  [unwired: 1 out]
          n378 = in-place-dvr #4(w834) -> (w842:cluster{dbl[], dbl[]}[][][])  [unwired: 1 out]
          n379 = in-place-dvr #5(w830) -> (w841:cluster{dbl[], dbl[]}[][][])  [unwired: 1 out]
          n380 = in-place-dvr #6(w831) -> (w840:cluster{dbl[], dbl[]}[][][])  [unwired: 1 out]
          n381 = in-place-dvr #7(w832) -> (w839:cluster{dbl[], dbl[]}[][][])  [unwired: 1 out]
          n382 = in-place-dvr #8(w833) -> (w838:cluster{dbl[], dbl[]}[][][])  [unwired: 1 out]
          n383 = Index Array(array=w843, index (dim 0)=w846) -> (element=w855:cluster{dbl[], dbl[]}[][])  [unwired: 2 in]
          n384 = Index Array(array=w842, index (dim 0)=w846) -> (element=w849:cluster{dbl[], dbl[]}[][])  [unwired: 2 in]
          n385 = Index Array(array=w841, index (dim 0)=w846, index (dim 1)=w844) -> (element=→"dV/dI 2T":cluster{dbl[], dbl[]}[])  [unwired: 1 in]
          n386 = Index Array(array=w840, index (dim 0)=w846) -> (element=w853:cluster{dbl[], dbl[]}[][])  [unwired: 2 in]
          n387 = Index Array(array=w839, index (dim 0)=w846, index (dim 1)=w844) -> (element=→"dV/dI":cluster{dbl[], dbl[]}[])  [unwired: 1 in]
          n388 = Index Array(array=w838, index (dim 0)=w846) -> (element=w851:cluster{dbl[], dbl[]}[][])  [unwired: 2 in]
          n389 = Index Array(array=w855, index (row)=w844) -> (element=→"IV":cluster{dbl[], dbl[]}[])  [unwired: 1 in]
          n390 = Index Array(array=w849, index (row)=w844) -> (element=→"dI/dV 2T":cluster{dbl[], dbl[]}[])  [unwired: 1 in]
          n391 = Index Array(array=w853, index (row)=w844) -> (element=→"dI/dV":cluster{dbl[], dbl[]}[])  [unwired: 1 in]
          n392 = Index Array(array=w851, index (row)=w844) -> (element=→"IV 2T":cluster{dbl[], dbl[]}[])  [unwired: 1 in]
          n393 = in-place-dvr #3(w843) -> ()  [unwired: 2 out]
          n394 = in-place-dvr #4(w842) -> ()  [unwired: 2 out]
          n395 = in-place-dvr #5(w841) -> ()  [unwired: 2 out]
          n396 = in-place-dvr #6(w840) -> ()  [unwired: 2 out]
          n397 = in-place-dvr #7(w839) -> ()  [unwired: 2 out]
          n398 = in-place-dvr #8(w838) -> ()  [unwired: 2 out]
        }
        n399 = call <vilib>:"Add State(s) to Queue__jki_lib_state_machine.vi"("State(s) in (\"\")"=w837) -> ("States Out"=w836:string)  [unwired: 14 in]
      }
      frame "Data Visualize: Vary Vslow" {
        # "col[]"
        # "row[]"
        # "page"
        # "Template Separator\n(You can make a copy of, or modify, this frame)"
        n400 = Unbundle By Name(w860) -> ("DVR"=w859:T18, "Page"=w856:i32, "Row Array"=w858:i32[], "Column Array"=w857:i32[])
        n401 = Unbundle By Name(w859) -> ("IV-4T"=w864:refnum<data-value>, "G-2T"=w863:refnum<data-value>, "G-4T"=w861:refnum<data-value>, "IV-2T"=w862:refnum<data-value>)
        n402 = in-place {
          in-place-border: w856 -> [w878]
          in-place-border: w858 -> [w873]
          in-place-border: w857 -> [w872]
          n403 = in-place-dvr #9(w864) -> (w871:cluster{dbl[], dbl[]}[][][])  [unwired: 1 out]
          n404 = in-place-dvr #10(w863) -> (w870:cluster{dbl[], dbl[]}[][][])  [unwired: 1 out]
          n405 = in-place-dvr #11(w861) -> (w869:cluster{dbl[], dbl[]}[][][])  [unwired: 1 out]
          n406 = in-place-dvr #12(w862) -> (w868:cluster{dbl[], dbl[]}[][][])  [unwired: 1 out]
          n407 = for {
            tunnel: w870 -> [w889]
            tunnel: w878 -> [w882]
            tunnel: w872 -> [w880] mode=indexing
            tunnel: [w888] -> w877 mode=indexing
            tunnel: w873 -> [w881] mode=indexing
            tunnel: w869 -> [w887]
            tunnel: [w886] -> w876 mode=indexing
            tunnel: w868 -> [w885]
            tunnel: [w884] -> w875 mode=indexing
            tunnel: w871 -> [w883]
            tunnel: [w879] -> w874 mode=indexing
            n408 = Index Array(array=w883, index (dim 0)=w882, index (dim 1)=w881, index (dim 2)=w880) -> (element=w879:cluster{dbl[], dbl[]})
            n409 = Index Array(array=w889, index (dim 0)=w882, index (dim 1)=w881, index (dim 2)=w880) -> (element=w888:cluster{dbl[], dbl[]})
            n410 = Index Array(array=w887, index (dim 0)=w882, index (dim 1)=w881, index (dim 2)=w880) -> (element=w886:cluster{dbl[], dbl[]})
            n411 = Index Array(array=w885, index (dim 0)=w882, index (dim 1)=w881, index (dim 2)=w880) -> (element=w884:cluster{dbl[], dbl[]})
          }
          "IV slow 4T" <- w874
          "dI/dV slow 4T" <- w876
          "dI/dV slow 2T" <- w877
          "IV slow 2T" <- w875
          n412 = in-place-dvr #9(w871) -> ()  [unwired: 2 out]
          n413 = in-place-dvr #10(w870) -> ()  [unwired: 2 out]
          n414 = in-place-dvr #11(w869) -> ()  [unwired: 2 out]
          n415 = in-place-dvr #12(w868) -> ()  [unwired: 2 out]
        }
        n416 = call <vilib>:"Add State(s) to Queue__jki_lib_state_machine.vi"("State(s) in (\"\")"=w867) -> ("States Out"=w866:string)  [unwired: 14 in]
      }
      frame "Data Visualize: Vary Fields" {
        # "column"
        # "row"
        # "Template Separator\n(You can make a copy of, or modify, this frame)"
        n417 = Unbundle By Name(w893) -> ("DVR"=w892:T18, "Row"=w891:i32, "Column"=w890:i32)
        n418 = Unbundle By Name(w892) -> ("IV-4T"=w894:refnum<data-value>, "G-2T"=w896:refnum<data-value>, "G-4T"=w895:refnum<data-value>, "IV-2T"=w897:refnum<data-value>)
        n419 = in-place {
          in-place-border: w891 -> [w901]
          in-place-border: w890 -> [w910]
          n420 = in-place-dvr #13(w894) -> (w905:cluster{dbl[], dbl[]}[][][])  [unwired: 1 out]
          n421 = in-place-dvr #14(w896) -> (w904:cluster{dbl[], dbl[]}[][][])  [unwired: 1 out]
          n422 = in-place-dvr #15(w895) -> (w903:cluster{dbl[], dbl[]}[][][])  [unwired: 1 out]
          n423 = in-place-dvr #16(w897) -> (w902:cluster{dbl[], dbl[]}[][][])  [unwired: 1 out]
          n424 = Index Array(array=w905, index (dim 1)=w901, index (dim 2)=w910) -> (element=→"IV vary 3rd 4T":cluster{dbl[], dbl[]}[])  [unwired: 1 in]
          n425 = Index Array(array=w904, index (dim 1)=w901, index (dim 2)=w910) -> (element=→"dI/dV vary 3rd 2T":cluster{dbl[], dbl[]}[])  [unwired: 1 in]
          n426 = Index Array(array=w903, index (dim 1)=w901, index (dim 2)=w910) -> (element=→"dI/dV vary 3rd 4T":cluster{dbl[], dbl[]}[])  [unwired: 1 in]
          n427 = Index Array(array=w902, index (dim 1)=w901, index (dim 2)=w910) -> (element=→"IV vary 3rd 2T":cluster{dbl[], dbl[]}[])  [unwired: 1 in]
          n428 = in-place-dvr #13(w905) -> ()  [unwired: 2 out]
          n429 = in-place-dvr #14(w904) -> ()  [unwired: 2 out]
          n430 = in-place-dvr #15(w903) -> ()  [unwired: 2 out]
          n431 = in-place-dvr #16(w902) -> ()  [unwired: 2 out]
        }
        n432 = call <vilib>:"Add State(s) to Queue__jki_lib_state_machine.vi"("State(s) in (\"\")"=w900) -> ("States Out"=w899:string)  [unwired: 14 in]
      }
      frame "Data Visualize: Choose Data 1" {
        # "Template Separator\n(You can make a copy of, or modify, this frame)"
        n433 = local read "Intensity 1"() -> (w922:T6)
        n434 = Unbundle By Name(w935) -> ("Vfast Slice"=w914:dbl[], "Graph.Intensity 1"=w930:refnum<class "graph_utilities.lvclass">, "DVR"=w934:T18, "Page"=w933:i32, "Row"=w931:i32)
        n435 = case shown="\"IV-2T\"" w922 {
          tunnel: w934 -> [w946 w948 w950 w952 w954 w956 w958]
          tunnel: [w945 w947 w949 w951 w953 w955 w957] -> w932
          frame "IV-4T", Default {
            n436 = Unbundle By Name(w946) -> ("IV-4T"=w945:refnum<data-value>)
          }
          frame "IV-2T" {
            n437 = Unbundle By Name(w948) -> ("IV-2T"=w947:refnum<data-value>)
          }
          frame "R-4T" {
            n438 = Unbundle By Name(w950) -> ("R-4T"=w949:refnum<data-value>)
          }
          frame "G-4T" {
            n439 = Unbundle By Name(w952) -> ("G-4T"=w951:refnum<data-value>)
          }
          frame "R-2T" {
            n440 = Unbundle By Name(w954) -> ("R-2T"=w953:refnum<data-value>)
          }
          frame "G-2T" {
            n441 = Unbundle By Name(w956) -> ("G-2T"=w955:refnum<data-value>)
          }
          frame "dGdVsg-4T" {
            n442 = Unbundle By Name(w958) -> ("G-4T"=w957:refnum<data-value>)
          }
        }
        n443 = call "Slice Row (DVR).vi"("Fake Point (0)"="fake point 1", "error in (no error)"=w915, "Row"=w931, "Page"=w933, "Data Value Reference in"=w932) -> ("X-array"=w913:dbl[], "2D Array"=w927:dbl[][])  [unwired: 4 in, 1 out]
        n444 = call "G to e2h (2D).vi"("e^2/h?"="e^2/h? 1", "Array in"=w927) -> ("error out"=w923:errorcluster, "Array out"=w928:dbl[][])  [unwired: 8 in]
        n445 = Subtract(x=w913, y="X Offset 1") -> (x-y=w911:dbl[])
        n446 = call "Log (2D).vi"("error in (no error)"=w923, "Log scale?"="Log scale? 1", "Array in"=w928) -> ("error out"=w924:errorcluster, "Array out"=w926:dbl[][])  [unwired: 7 in]
        n447 = case shown="\"dGdVsg-4T\"" w922 {
          tunnel: w926 -> [w939 w944]
          tunnel: [w939 w943] -> w925
          tunnel: w924 -> [w938 w942]
          tunnel: [w938 w941] -> w919
          tunnel: w914 -> [_ w940]
          frame Default {
          }
          frame "dGdVsg-4T" {
            n448 = call "Derivative (2D).vi"("error in (no error)"=w942, "Axis Array"=w940, "Conductance"=w944) -> ("error out"=w941:errorcluster, "Transconductance"=w943:dbl[][])  [unwired: 6 in, 1 out]
          }
        }
        n449 = call <userlib>:"Set Intensity Graph Value.vi"("error in (no error)"=w919, "Value"=w925, "graph_utilities in"=w930) -> ("error out"=w918:errorcluster, "graph_utilities out"=w929:refnum<class "graph_utilities.lvclass">)  [unwired: 7 in]
        n450 = call <userlib>:"Set Intensity Graph X Scale Array.vi"("error in (no error)"=w918, "X Scale"=w911, "graph_utilities in"=w929) -> ("error out"=w917:errorcluster)  [unwired: 7 in, 1 out]
        n451 = call <vilib>:"Add State(s) to Queue__jki_lib_state_machine.vi"("State(s) in (\"\")"=w937) -> ("States Out"=w936:string)  [unwired: 14 in]
      }
      frame "Data Visualize: Choose Data 2" {
        # "Template Separator\n(You can make a copy of, or modify, this frame)"
        n452 = Unbundle By Name(w983) -> ("Vfast Slice"=w962:dbl[], "Graph.Intensity 2"=w978:refnum<class "graph_utilities.lvclass">, "DVR"=w982:T18, "Page"=w981:i32, "Row"=w979:i32)
        n453 = local read "Intensity 2"() -> (w963:T6)
        n454 = case shown="\"dGdVsg-4T\"" w963 {
          tunnel: w982 -> [w994 w996 w998 w1000 w1002 w1004 w1006]
          tunnel: [w993 w995 w997 w999 w1001 w1003 w1005] -> w980
          frame "IV-4T", Default {
            n455 = Unbundle By Name(w994) -> ("IV-4T"=w993:refnum<data-value>)
          }
          frame "IV-2T" {
            n456 = Unbundle By Name(w996) -> ("IV-2T"=w995:refnum<data-value>)
          }
          frame "R-4T" {
            n457 = Unbundle By Name(w998) -> ("R-4T"=w997:refnum<data-value>)
          }
          frame "G-4T" {
            n458 = Unbundle By Name(w1000) -> ("G-4T"=w999:refnum<data-value>)
          }
          frame "R-2T" {
            n459 = Unbundle By Name(w1002) -> ("R-2T"=w1001:refnum<data-value>)
          }
          frame "G-2T" {
            n460 = Unbundle By Name(w1004) -> ("G-2T"=w1003:refnum<data-value>)
          }
          frame "dGdVsg-4T" {
            n461 = Unbundle By Name(w1006) -> ("G-4T"=w1005:refnum<data-value>)
          }
        }
        n462 = call "Slice Row (DVR).vi"("Fake Point (0)"="fake point 2", "error in (no error)"=w964, "Row"=w979, "Page"=w981, "Data Value Reference in"=w980) -> ("X-array"=w961:dbl[], "2D Array"=w975:dbl[][])  [unwired: 4 in, 1 out]
        n463 = call "G to e2h (2D).vi"("e^2/h?"="e^2/h? 2", "Array in"=w975) -> ("error out"=w971:errorcluster, "Array out"=w976:dbl[][])  [unwired: 8 in]
        n464 = Subtract(x=w961, y="X Offset 2") -> (x-y=w960:dbl[])
        n465 = call "Log (2D).vi"("error in (no error)"=w971, "Log scale?"="Log scale? 2", "Array in"=w976) -> ("error out"=w972:errorcluster, "Array out"=w974:dbl[][])  [unwired: 7 in]
        n466 = case shown="\"dGdVsg-4T\"" w963 {
          tunnel: w974 -> [w987 w992]
          tunnel: [w987 w991] -> w973
          tunnel: w972 -> [w986 w990]
          tunnel: [w986 w989] -> w968
          tunnel: w962 -> [_ w988]
          frame Default {
          }
          frame "dGdVsg-4T" {
            n467 = call "Derivative (2D).vi"("error in (no error)"=w990, "Axis Array"=w988, "Conductance"=w992) -> ("error out"=w989:errorcluster, "Transconductance"=w991:dbl[][])  [unwired: 6 in, 1 out]
          }
        }
        n468 = call <userlib>:"Set Intensity Graph Value.vi"("error in (no error)"=w968, "Value"=w973, "graph_utilities in"=w978) -> ("error out"=w967:errorcluster, "graph_utilities out"=w977:refnum<class "graph_utilities.lvclass">)  [unwired: 7 in]
        n469 = call <userlib>:"Set Intensity Graph X Scale Array.vi"("error in (no error)"=w967, "X Scale"=w960, "graph_utilities in"=w977) -> ("error out"=w966:errorcluster)  [unwired: 7 in, 1 out]
        n470 = call <vilib>:"Add State(s) to Queue__jki_lib_state_machine.vi"("State(s) in (\"\")"=w985) -> ("States Out"=w984:string)  [unwired: 14 in]
      }
      frame "---------- Data Export ----------" {
        # "Template Separator\n(You can make a copy of, or modify, this frame)"
        n471 = call <vilib>:"Add State(s) to Queue__jki_lib_state_machine.vi"("State(s) in (\"\")"=w1010) -> ("States Out"=w1009:string)  [unwired: 14 in]
      }
      frame "Data Export: Export" {
        # "Template Separator\n(You can make a copy of, or modify, this frame)"
        n472 = Unbundle By Name(w1017) -> ("Graph"=w1016:T17)
        n473 = case shown="\"Intensity 1\", Default" "Export What?" {
          selector: "Export What?" -> [w1020 w1034 w1051 w1067 w1086 w1105]
          tunnel: w1016 -> [w1032 w1049 w1066 w1079 w1096 w1113]
          tunnel: w1013 -> [w1029 w1039 w1058 w1075 w1082 w1098]
          tunnel: [w1027 w1046 w1063 w1074 w1093 w1110] -> w1015
          tunnel: "Export ITX Path" -> [w1024 w1037 w1054 w1069 w1092 w1104]
          tunnel: "Export ITX Name" -> [w1023 w1038 w1053 w1070 w1088 w1107]
          frame "Intensity 1", Default {
            n474 = local read "Intensity 1"() -> (w1021:T6)
            n475 = Format Into String(format string="%s-%s-%s-", w1023, w1021, w1020) -> (resulting string=w1026:string)  [unwired: 2 in, 1 out]
            n476 = Unbundle By Name(w1032) -> ("Intensity 1"=w1031:refnum<class "graph_utilities.lvclass">)
            n477 = Build Path(base path=w1024, name or relative path=w1026) -> (appended path=w1022:path)
            n478 = call <userlib>:"Read Intensity Graph ref.vi"("error in (no error)"=w1029, "graph_utilities in"=w1031) -> ("error out"=w1028:errorcluster, "Intensity Graph"=w1030:refnum<vi>)  [unwired: 6 in, 2 out]
            n479 = call <userlib>:"Intensity Graph to Igor Graph.vi"("error in (no error)"=w1028, "Intensity Graph Reference"=w1030, "Path"=w1022) -> ("error out"=w1027:errorcluster)  [unwired: 7 in, 1 out]
          }
          frame "H Cut 1" {
            n480 = local read "Intensity 1"() -> (w1033:T6)
            n481 = Unbundle By Name(w1049) -> ("H 1"=w1042:refnum<class "graph_utilities.lvclass">)
            n482 = call <userlib>:"Get Intensity Graph Cursor (Control).vi"("error in (no error)"=w1039, "graph_utilities in"=w1042) -> ("error out"=w1040:errorcluster, "Cursor.Cursor Position"=w1043:T21, "graph_utilities out"=w1041:refnum<class "graph_utilities.lvclass">)  [unwired: 7 in]
            n483 = Unbundle By Name(w1043) -> ("Y"=w1035:dbl)
            n484 = Format Into String(format string="%s-%s-%s-%f-", w1038, w1033, w1034, w1035) -> (resulting string=w1045:string)  [unwired: 2 in, 1 out]
            n485 = call <userlib>:"Read XY Graph ref.vi"("error in (no error)"=w1040, "graph_utilities in"=w1041) -> ("error out"=w1048:errorcluster, "XY Graph"=w1047:refnum<vi>)  [unwired: 6 in, 2 out]
            n486 = Build Path(base path=w1037, name or relative path=w1045) -> (appended path=w1036:path)
            n487 = call <userlib>:"XY Graph to Igor Graph.vi"("error in (no error)"=w1048, "XY Graph Reference"=w1047, "Path"=w1036) -> ("error out"=w1046:errorcluster)  [unwired: 7 in, 1 out]
          }
          frame "V Cut 1" {
            n488 = local read "Intensity 1"() -> (w1050:T6)
            n489 = Unbundle By Name(w1066) -> ("V 1"=w1059:refnum<class "graph_utilities.lvclass">)
            n490 = call <userlib>:"Get Intensity Graph Cursor (Control).vi"("error in (no error)"=w1058, "graph_utilities in"=w1059) -> ("error out"=w1056:errorcluster, "Cursor.Cursor Position"=w1060:T21, "graph_utilities out"=w1057:refnum<class "graph_utilities.lvclass">)  [unwired: 7 in]
            n491 = Unbundle By Name(w1060) -> ("X"=w1052:dbl)
            n492 = Format Into String(format string="%s-%s-%s-%f-", w1053, w1050, w1051, w1052) -> (resulting string=w1062:string)  [unwired: 2 in, 1 out]
            n493 = call <userlib>:"Read XY Graph ref.vi"("error in (no error)"=w1056, "graph_utilities in"=w1057) -> ("error out"=w1065:errorcluster, "XY Graph"=w1064:refnum<vi>)  [unwired: 6 in, 2 out]
            n494 = Build Path(base path=w1054, name or relative path=w1062) -> (appended path=w1055:path)
            n495 = call <userlib>:"XY Graph to Igor Graph.vi"("error in (no error)"=w1065, "XY Graph Reference"=w1064, "Path"=w1055) -> ("error out"=w1063:errorcluster)  [unwired: 7 in, 1 out]
          }
          frame "Intensity 2" {
            n496 = local read "Intensity 2"() -> (w1071:T6)
            n497 = Format Into String(format string="%s-%s-%s-", w1070, w1071, w1067) -> (resulting string=w1073:string)  [unwired: 2 in, 1 out]
            n498 = Unbundle By Name(w1079) -> ("Intensity 2"=w1076:refnum<class "graph_utilities.lvclass">)
            n499 = Build Path(base path=w1069, name or relative path=w1073) -> (appended path=w1068:path)
            n500 = call <userlib>:"Read Intensity Graph ref.vi"("error in (no error)"=w1075, "graph_utilities in"=w1076) -> ("error out"=w1077:errorcluster, "Intensity Graph"=w1078:refnum<vi>)  [unwired: 6 in, 2 out]
            n501 = call <userlib>:"Intensity Graph to Igor Graph.vi"("error in (no error)"=w1077, "Intensity Graph Reference"=w1078, "Path"=w1068) -> ("error out"=w1074:errorcluster)  [unwired: 7 in, 1 out]
          }
          frame "H Cut 2" {
            n502 = local read "Intensity 2"() -> (w1087:T6)
            n503 = Unbundle By Name(w1096) -> ("H 2"=w1084:refnum<class "graph_utilities.lvclass">)
            n504 = call <userlib>:"Get Intensity Graph Cursor (Control).vi"("error in (no error)"=w1082, "graph_utilities in"=w1084) -> ("error out"=w1081:errorcluster, "Cursor.Cursor Position"=w1085:T21, "graph_utilities out"=w1083:refnum<class "graph_utilities.lvclass">)  [unwired: 7 in]
            n505 = Unbundle By Name(w1085) -> ("Y"=w1080:dbl)
            n506 = Format Into String(format string="%s-%s-%s-%f-", w1088, w1087, w1086, w1080) -> (resulting string=w1091:string)  [unwired: 2 in, 1 out]
            n507 = call <userlib>:"Read XY Graph ref.vi"("error in (no error)"=w1081, "graph_utilities in"=w1083) -> ("error out"=w1095:errorcluster, "XY Graph"=w1094:refnum<vi>)  [unwired: 6 in, 2 out]
            n508 = Build Path(base path=w1092, name or relative path=w1091) -> (appended path=w1089:path)
            n509 = call <userlib>:"XY Graph to Igor Graph.vi"("error in (no error)"=w1095, "XY Graph Reference"=w1094, "Path"=w1089) -> ("error out"=w1093:errorcluster)  [unwired: 7 in, 1 out]
          }
          frame "V Cut 2" {
            n510 = local read "Intensity 2"() -> (w1106:T6)
            n511 = Unbundle By Name(w1113) -> ("V 2"=w1101:refnum<class "graph_utilities.lvclass">)
            n512 = call <userlib>:"Get Intensity Graph Cursor (Control).vi"("error in (no error)"=w1098, "graph_utilities in"=w1101) -> ("error out"=w1099:errorcluster, "Cursor.Cursor Position"=w1102:T21, "graph_utilities out"=w1100:refnum<class "graph_utilities.lvclass">)  [unwired: 7 in]
            n513 = Unbundle By Name(w1102) -> ("X"=w1097:dbl)
            n514 = Format Into String(format string="%s-%s-%s-%f-", w1107, w1106, w1105, w1097) -> (resulting string=w1109:string)  [unwired: 2 in, 1 out]
            n515 = call <userlib>:"Read XY Graph ref.vi"("error in (no error)"=w1099, "graph_utilities in"=w1100) -> ("error out"=w1112:errorcluster, "XY Graph"=w1111:refnum<vi>)  [unwired: 6 in, 2 out]
            n516 = Build Path(base path=w1104, name or relative path=w1109) -> (appended path=w1103:path)
            n517 = call <userlib>:"XY Graph to Igor Graph.vi"("error in (no error)"=w1112, "XY Graph Reference"=w1111, "Path"=w1103) -> ("error out"=w1110:errorcluster)  [unwired: 7 in, 1 out]
          }
        }
        n518 = call <vilib>:"Add State(s) to Queue__jki_lib_state_machine.vi"("State(s) in (\"\")"=w1019) -> ("States Out"=w1018:string)  [unwired: 14 in]
      }
    }
  }
